vi "WHD_VEten_0.1.1_WS_BIDIR.vi"() -> ()   [LabVIEW 2015]
uses:
  <vilib>/LabVIEW Targets/FPGA/cRIO/shared/nicrio_ModuleControls/nicrio_cRIO-9234_DataRatesRing2.ctl
  <vilib>/RTwatchdog.llb/Watchdog expiration actions.ctl
  <vilib>/userDefined/High Color/nirio_resource_hc.ctl
  <vilib>/FPGAPlugInAG/cRIO-9031/niLvFpga_Open_cRIO-9031.vi
  <vilib>/Utility/error.llb/Error Cluster From Error Code.vi
  <vilib>/rvi/errors/niLvFpgaAdjustHostInterfaceError.vi
  <vilib>/Utility/file.llb/Write Delimited Spreadsheet (string).vi
  <vilib>/FPGAPlugInAG/cRIO-9031/niLvFpga_Run_cRIO-9031.vi
  <vilib>/rvi/interface/common/niFpgaWaitOnOcc.vi
  <vilib>/FPGAPlugInAG/cRIO-9031/niLvFpga_Reset_cRIO-9031.vi
  <vilib>/FPGAPlugInAG/cRIO-9031/niLvFpga_Close_cRIO-9031.vi
  <vilib>/rvi/interface/nirviOpenFPGA/nirviOpenFPGA.xnode
  FPGA Bitfiles/W&RDEuskotrenViz_FPGATarget2_FPGA8a2wsBIdirec_eiRvK+Hs3vw.lvbitx
  <vilib>/rvi/interface/nirviReadWriteControl/nirviReadWriteControl.xnode
  <vilib>/rvi/interface/nirviMethod/nirviMethod.xnode
  <vilib>/rvi/interface/nirviCloseFPGA/nirviCloseFPGA.xnode
  <vilib>/NI_Real-Time Target Support.lvlib
  <vilib>/rvi/errors/niLvFpgaMergeErrorWithErrorCode.vi
  <vilib>/nisyscfg/nisyscfg.lvlib
  AURA_Wheel/Json2Labv.lvlib
  AURA_Wheel/AuraWheelAPI/AuraWheel.lvlib
  NiFpgaLv.dll
  <vilib>/FPGAPlugInAG/cRIO-9031/niLvFpga_ConfigureFifo_cRIO-9031.vi
  <vilib>/FPGAPlugInAG/cRIO-9031/niLvFpga_StartFifo_cRIO-9031.vi
  <vilib>/FPGAPlugInAG/cRIO-9031/niLvFpga_ReadFifo_cRIO-9031.vi
  <vilib>/FPGAPlugInAG/cRIO-9031/niLvFpga_StopFifo_cRIO-9031.vi
panel:
  out "Direccion 0?":bool
  out "Boton Adquirir?":bool
  out "RuedaDetectada2?":bool=TRUE
  out "RuedaDetectada1?":bool=TRUE
  in  "Timeout ruedas":dbl
  in  "Borrar archivos\nadquisicion con error":bool
  in  "Able watchdog?":bool
  in  "Reset watchdog?":bool
  in  "Leer config RFID NEM":bool
  in  "bytes to read":i32
  in  "DeviceAddress":u8
  in  "timeout ms (60000)":i32
  in  "Max archivos":u32=2
  in  "Bytes libre despues de borrar":u32=2
  in  "Bytes min libre":u32=2
  in  "Nº de acelerómetros":i32
  in  "Nº inductivos":i32
  in  "Offset_rueda WS 1":fxp<+/-,24,-4>=0.004999998956918716 format="%.27g"
  out "TAGs_AURAwheel":string[][](array[string])
  out "Plataformas?":bool
  out "Nº Ejes":i32[](array[numeric])
  out "Nº UTs":i32
  out "it-read-LR6":i32[](array[numeric])
  out "it-LR6":i32
  out "RFID_LR6_Error":errorcluster
  out "Series_flota":string[](array[string])
  out "Tabla_flota":string[][](array[string])
  out "Puntos medios de las ventanas":dbl[][](array[numeric])
  out "configuration file path":path=path "c:/Parametros.cfg"
  in  "IP synchr":string
  out "data":cluster{"status":string}
  out "confRFID":path=path "c:/RFID/TAGS.csv"
  out "TAGS leidos":path=path "c:/RFID/TAGS.csv"
  in  "Use Aura?":bool
  in  "Parametros AuraWheel":string[](array[string])
  in  "Parámetros acelerómetros":dbl[](array[numeric])
  in  "Tiempo de adquisicion":dbl=10.0
  in  "Adquirir":bool
  out "Fin":bool
  out "Contador":i32=1
  out "Path TEST":path=path "c:/TEST"
  out "Fallo fotocelula":bool
  out "Path_Borrar":path=path "c:/Trenes"
  out "Longitud de la unidad":dbl
  out "Aviso no detección":string
  out "Time to Acquire Block (ms)":i32
  out "Distancia de acelerómetros":dbl[](array[numeric])
  out "Block Size":u32
  out "Distancias generales":dbl[](array[numeric])
  in  "Reset del controlador":bool
  in  "Configuración":bool
  in  "Parar la aplicación":bool
  out "RFID":bool=TRUE
  out "date/time string":string
  out "Timeout ruedas":bool
  out "Tiempo":dbl
  out "Inicio pasada":timestamp
  out "Ultimo TEST":timestamp
  out "Fuente":bool=TRUE
  out "Estado":string
  out "RFID_ID":refnum<k5>
  out "DC OK":string
  out "Aviso temperatura":string
  in  "Tab Control":T1(tab)=enum."Parámetros"
  out "V (m/s)":dbl
  out "Temperatura (ºC)":dbl
  out "Max RMS Ruedas":dbl[][](array[numeric])
  out "result":bool
  out "TAGs":string[](array[string])
  out "Parar":bool
  out "TAGs LR6":string[](array[string])
  out "TAGs HEX":string[](array[string])
  out "Waveform Graph 2":sgl[](graph)
  out "Waveform Graph":sgl[][](graph)
  out "Nombre de archivo":path[](array[path])
  out "Tiempo de paso (s)":dbl
  out "Tiempo extra de adquisición (s)":dbl
  out "Número de ejes detectados":i32
  out "Buffer Underflow":bool
  out "Buffer Overflow":bool
  out "Disco Duro Disponible (bytes)":i64
  out "created path":path
  out "Nº Ruedas 1":i32
  out "NºRuedas 2":i32
  out "deleted portion":sgl[](array[numeric])
  out "deleted portion 2":sgl[](array[numeric])
  out "Ejes_convoy":i32
  out "Archivo\nvalido?":bool
  out "T fuera rango":bool
  in  "Frecuencia de muestreo (Hz)":dbl=25600.0
  in  "Escaneos de la FIFO por canal":u32=5000
  in  "Tiempo extra al detector de paso (s)":dbl=1.0
  in  "dt RMS":dbl=256.0
  in  "Frecuencia de muestreo y módulo CRIO":T2=2 items=["51.200 kS/s (NI 9234)"=1, "25.600 kS/s (NI 9234)"=2, "17.067 kS/s (NI 9234)"=3, "12.800 kS/s (NI 9234)"=4, "10.240 kS/s (NI 9234)"=5, "8.533 kS/s (NI 9234)"=6, "7.314 kS/s (NI 9234)"=7, "6.400 kS/s (NI 9234)"=8, "5.689 kS/s (NI 9234)"=9, "5.120 kS/s (NI 9234)"=10, "4.654 kS/s (NI 9234)"=11, "4.267 kS/s (NI 9234)"=12, "3.938 kS/s (NI 9234)"=13, "3.657 kS/s (NI 9234)"=14, "3.413 kS/s (NI 9234)"=15, "3.200 kS/s (NI 9234)"=16, "3.012 kS/s (NI 9234)"=17, "2.845 kS/s (NI 9234)"=18, "2.695 kS/s (NI 9234)"=19, "2.560 kS/s (NI 9234)"=20, "2.438 kS/s (NI 9234)"=21, "2.328 kS/s (NI 9234)"=22, "2.226 kS/s (NI 9234)"=23, "2.133 kS/s (NI 9234)"=24, "2.048 kS/s (NI 9234)"=25, "1.969 kS/s (NI 9234)"=26, "1.896 kS/s (NI 9234)"=27, "1.829 kS/s (NI 9234)"=28, "1.765 kS/s (NI 9234)"=29, "1.707 kS/s (NI 9234)"=30, "1.652 kS/s (NI 9234)"=31]
  in  "Puerto RFID":u16=2189
  in  "IP RFID":string="192.168.106.99"
  in  "Offset_rueda WS 2":fxp<+/-,24,-4>=0.004999998956918716 format="%.27g"
  in  "Count(mSec)":u32=2
  in  "LR6 IP address":string="192.168.106.94"
  in  "Port LR6":u16=2001
  in  "RFID NEM on?":bool
  in  "RFID LR6 on?":bool
  in  "Canal cero WS1?":bool
  in  "Canal cero WS2":bool
  out "Parámetros":bool=TRUE
  out "Distacias y medidas de dispositivos":bool=TRUE
  out "RFID_Error":errorcluster
  out "error FPGA":errorcluster
  out "error manipulacion archivos":errorcluster
  out "Unidades y ejes":bool=TRUE
  out "RFID":bool=TRUE
  out "error AURA":errorcluster
  out "Response headers":string
  out "Numeric 3":i32
  in  "Digital?":bool=TRUE
  out "Bucle Espera":i32
  out "Watchdog config":T3={"reset"=FALSE, "occurrence"=FALSE, "trigger protocol"=enum."active high", "trigger line"=enum."none", "disable watchdog on VI exit"=TRUE}
  # "Funciona?"
  # "Última detección de unidad"
  # "Error!!"
  # "Estado de la memoria"
  # "Parámetros de muestreo"
  # "Parámetros de adquisición"
  # "Parámetros de procesado"
  # "Cambio Fecha y Hora"
  # "Cargar datos de configuración"
  # "Errores!!"
  # "WRD_MEX\nWRD_ZAR"
  # "0 tagMexInit\n1 tagMexFin\n\n0 tag1\n1 tag2"
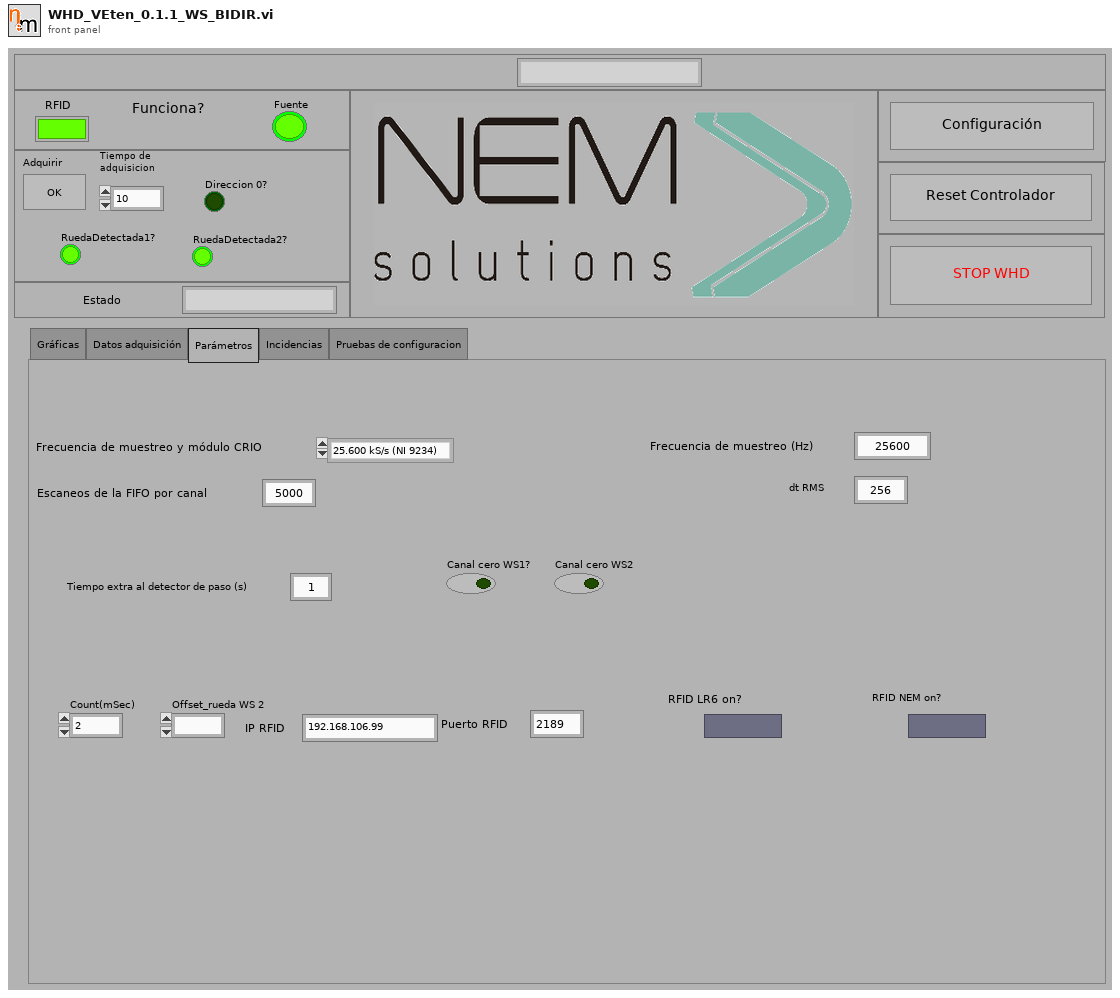
[diagram p1: front panel]
types:
  T1 = enum32{"Gráficas", "Datos adquisición", "Parámetros", "Incidencias", "Pruebas de configuracion"}
  T2 = typedef "nicrio_cRIO-9234_DataRatesRing2.ctl" = u8
  T3 = typedef "Watchdog expiration actions.ctl" = cluster{"reset":bool, "occurrence":bool, "trigger protocol":enum16{"active high", "active low", "open collector"}, "trigger line":enum16{"none", "line 0", "line 1", "line 2", "line 3", "line 4", "line 5", "line 6", "line 7", "SMB line 0"}, "disable watchdog on VI exit":bool}
  T4 = typedef "nirio_resource_hc.ctl" = tag
  T5 = enum16{"Standard", "Buffered", "CRLF", "Immediate"}
  T6 = enum16{"open", "replace", "create", "open or create", "replace or create", "replace or create with confirmation"}
  T7 = enum16{"big-endian, network order", "native, host order", "little-endian"}
  T8 = cluster{"error IO":errorcluster, bool[], u32[], string[], dbl[]}
  T9 = cluster{"g_ts":dbl, "p_sp":dbl, "p_tp":dbl, "p_tg":cluster{"tg_n":dbl, "tg_t":string}[], "p_ax":cluster{"ax_n":dbl, "ax_sp":dbl, "ax_wh":cluster{"wh_p":dbl, "wh_a1":dbl, "wh_a2":dbl, "wh_a3":dbl, "wh_a4":dbl}[]}[]}
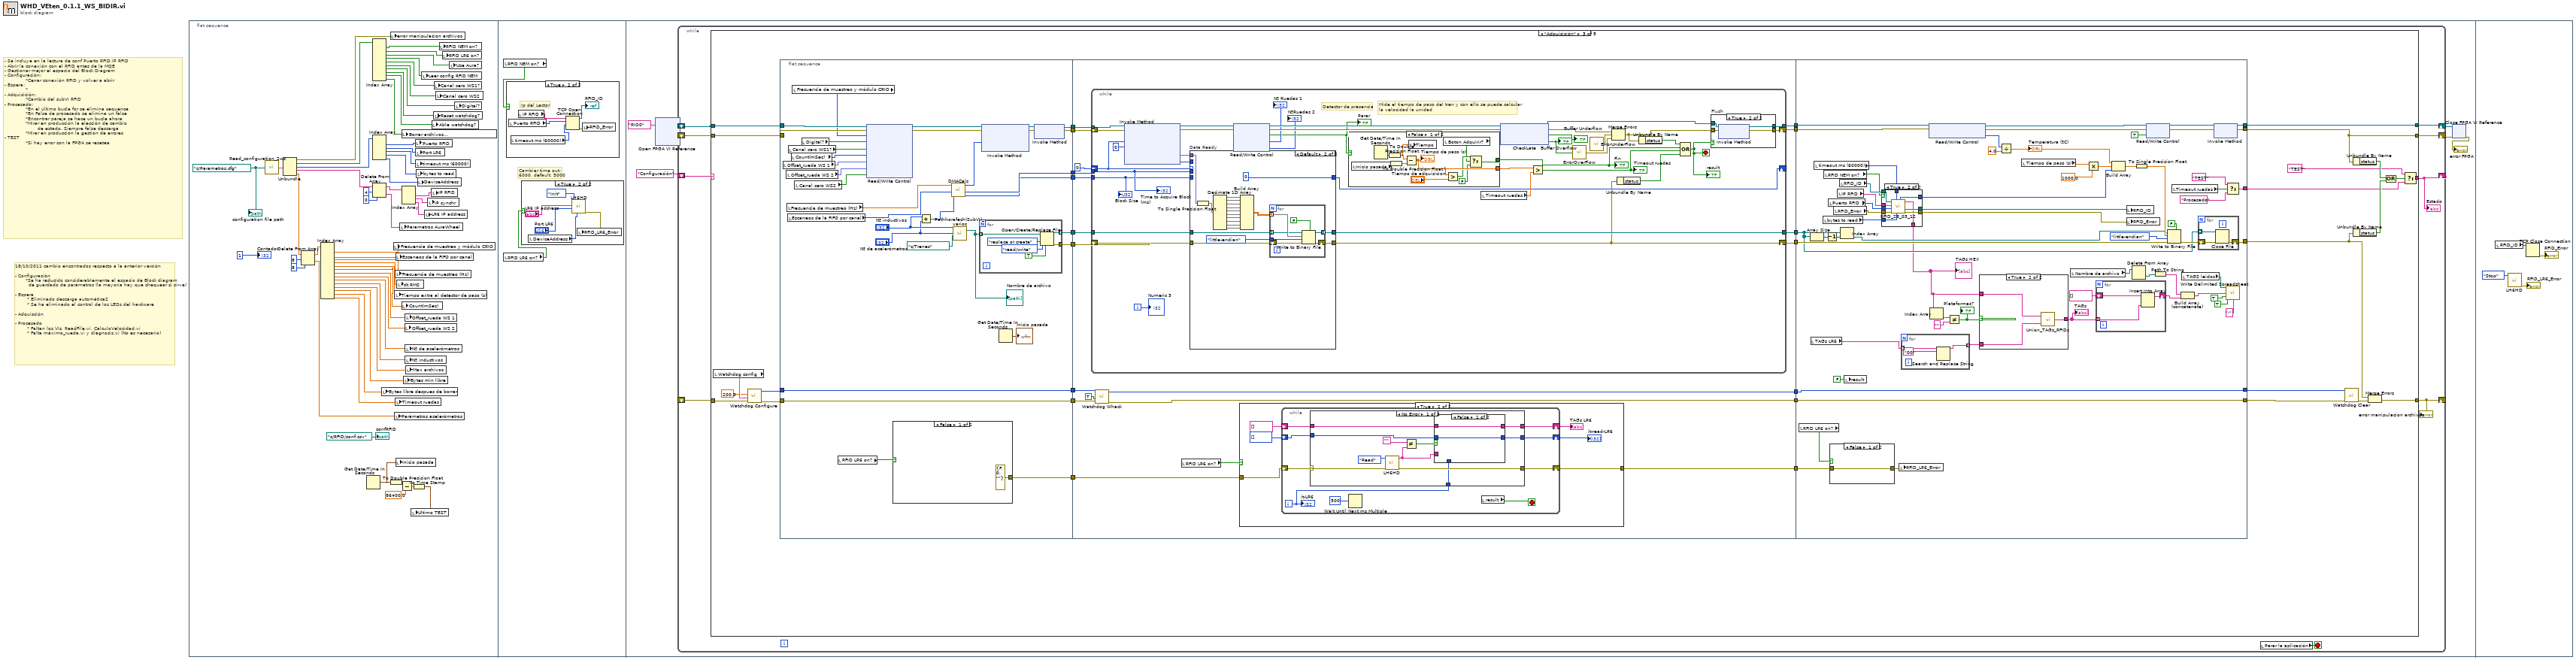
[diagram p0: block diagram]
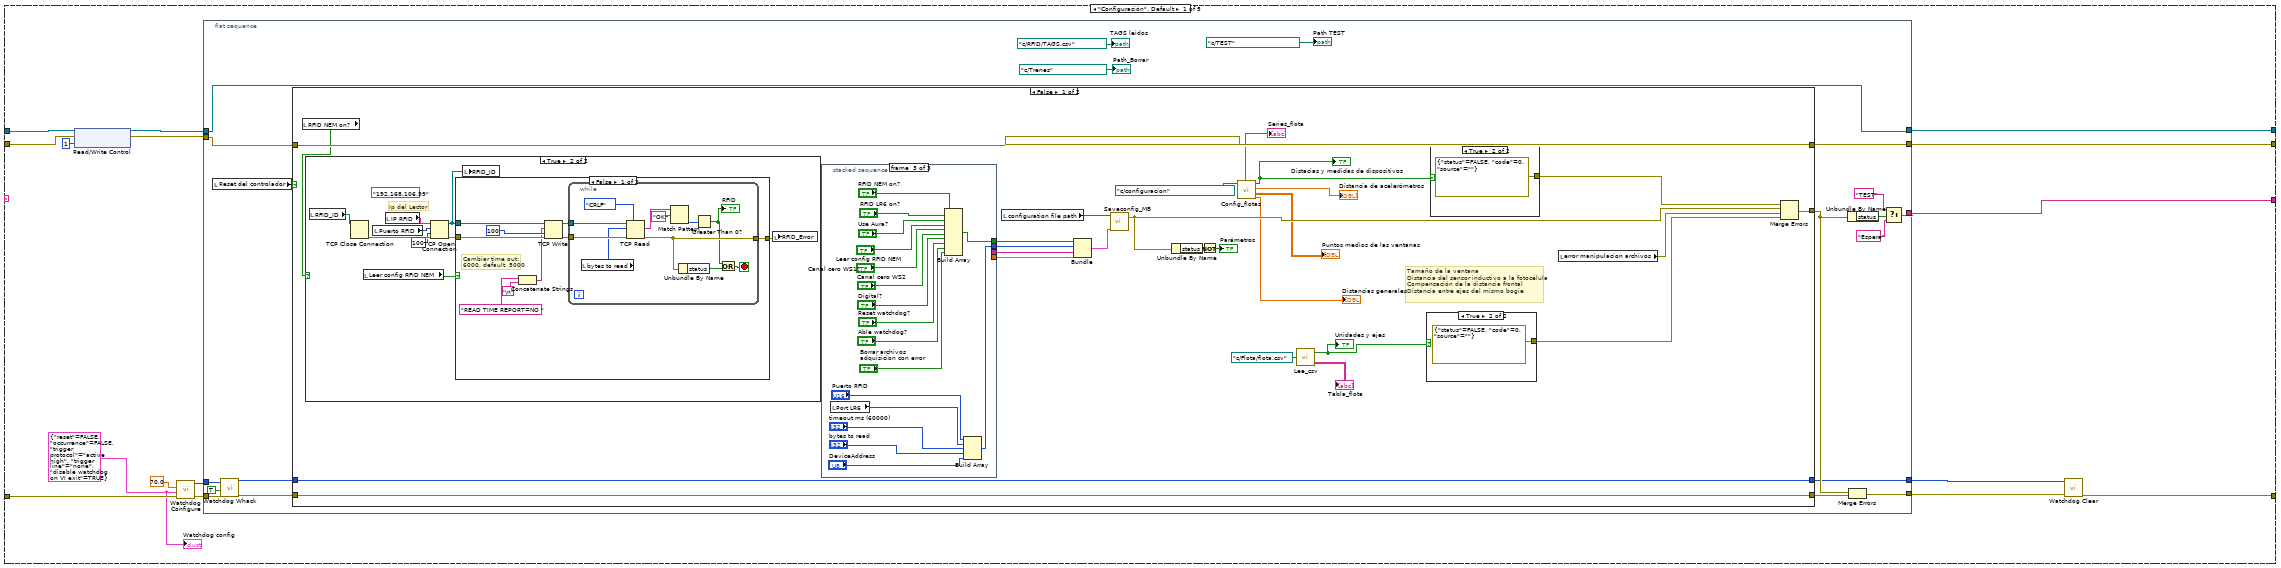
[diagram p4: hidden frame]
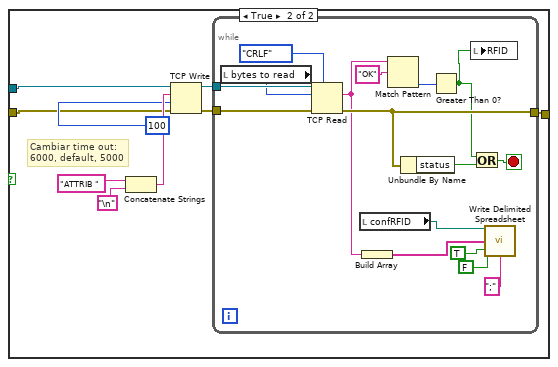
[diagram p6: hidden frame]
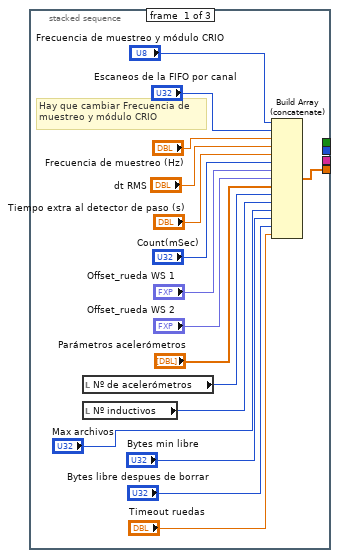
[diagram p7: hidden frame]
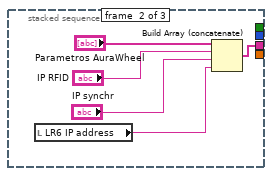
[diagram p8: hidden frame]
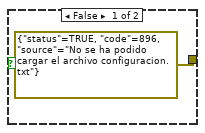
[diagram p9: hidden frame]
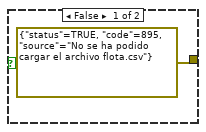
[diagram p10: hidden frame]
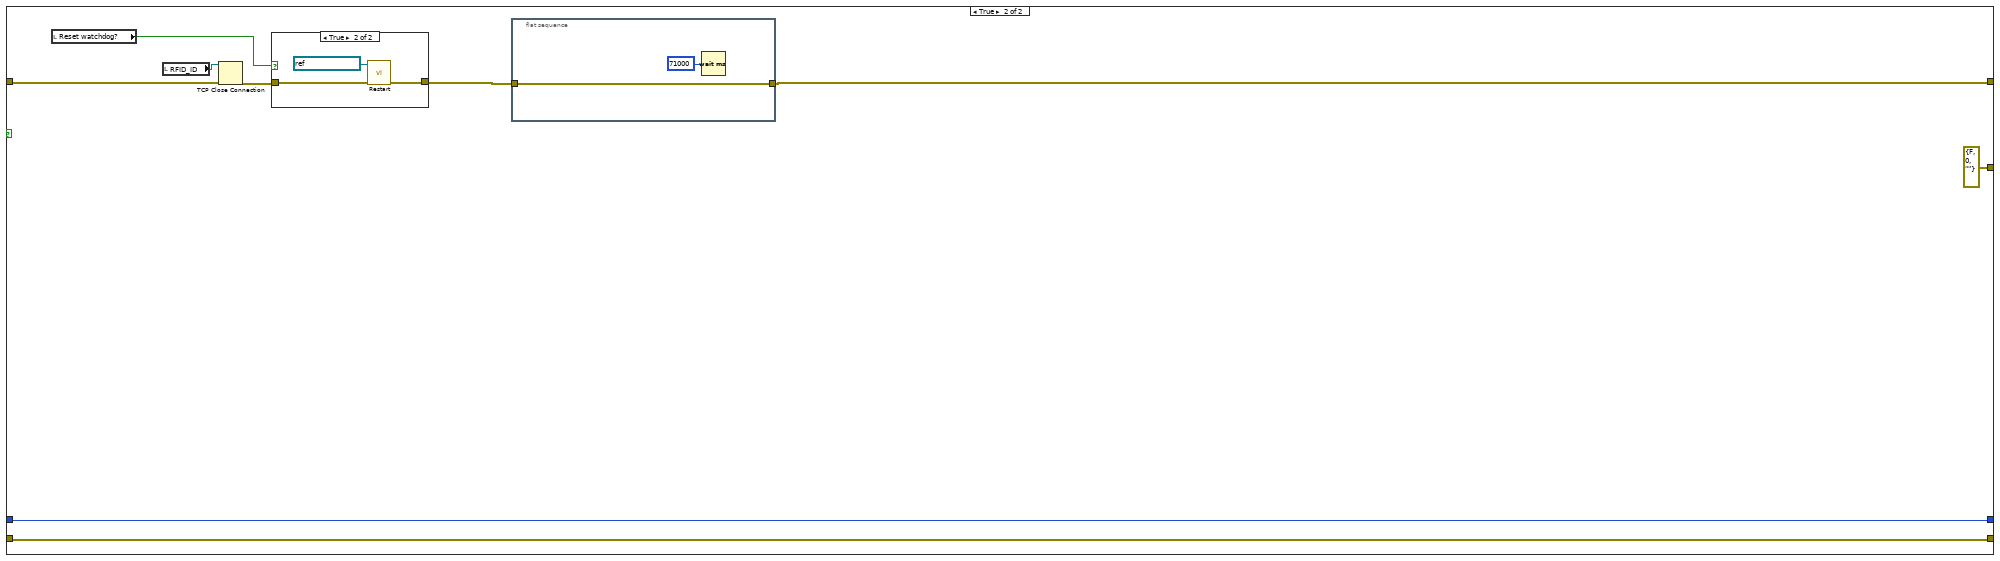
[diagram p11: hidden frame]
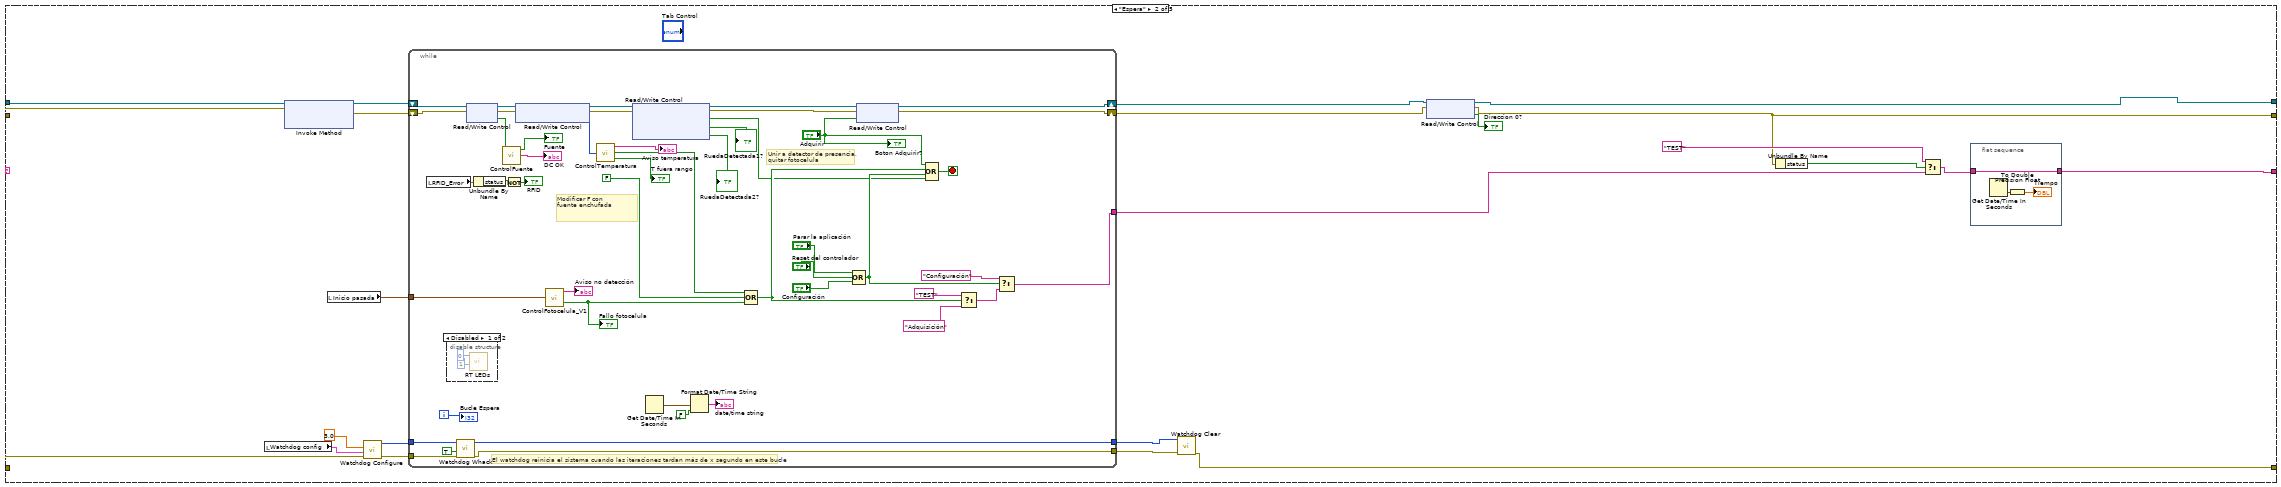
[diagram p13: hidden frame]
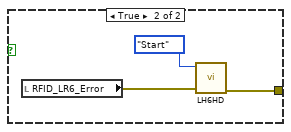
[diagram p15: hidden frame]
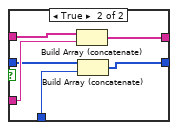
[diagram p17: hidden frame]
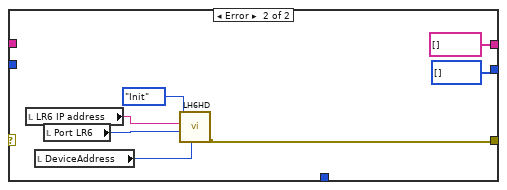
[diagram p18: hidden frame]
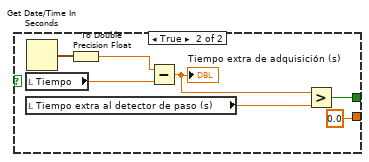
[diagram p19: hidden frame]
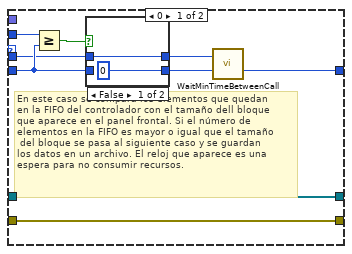
[diagram p20: hidden frame]
diagram:
  # "18/10/2011 cambio encontrados respecto a la anterior versión\n\n- Configuración\n       *Se ha reducido considerablemente el espacio de Block diagram\n         de guardado de parámetros (la mayoría hay que chequear si sirve)\n\n- Espera\n        * Eliminado descarga automática2\n        * Se ha eliminado el control de los LEDs del hardware\n       \n- Adquisción\n\n- Procesado\n        * Faltan los VIs, ReadFile.vi, CalculoVelocidad.vi\n        * Falta máximo_rueda.vi y diagnosis.vi (No es necesario)"
  # "- Se incluye en la lectura de conf Puerto RFID,IP RFID\n- Abrir la conexión con el RFID antes de la MQE\n- Gestionar mejor el espacio del Block Diagram\n- Configuración:\n              *Cerrar conexión RFID y volver a abrir\n- Espera:\n              *\n- Adquisición:\n              *Cambio del subVI RFID\n- Procesado:\n              *En el último bucle for se elimina sequence\n              *En False de procesado se elimina un false\n              *Encontrar pareja se hace un bucle ahora\n              *Mirar en producción la elección de cambio\n                      de estado. Siempre false descarga \n              *Mirar en produccion la gestion de errores\n- TEST\n              *Si hay error con la FPGA se resetea"
  n1 = flat-sequence {
    frame #0 {
      w38 = path "c:/Parametros.cfg" ("configuration file path")
      n2 = call "Read_configuration_2ws.vi"("configuration file path"=w38) -> ("output cluster"=w37:T8)
      n3 = Unbundle(w37) -> ("error IO"=w42:errorcluster, w41:bool[], w40:u32[], w29:string[], w35:dbl[])
      n4 = Delete From Array(array=w35, length=8, index=8) -> (deleted portion=w31:dbl[], array with subset deleted=w34:dbl[])
      n5 = Index Array(array=w34) -> (element #1=w49:dbl, element #2=w48:dbl, element #3=w47:dbl, element #4=w46:dbl, element #5=w45:dbl, element #6=w19:dbl, element #7=w18:dbl, element #8=w1:dbl, element #9=w17:dbl, element #10=w16:dbl, element #11=w15:dbl, element #12=w14:dbl, element #13=w13:dbl, element #14=w2:dbl)  [unwired: 14 in]
      n6 = Get Date/Time In Seconds() -> (seconds since 1Jan1904=w51:timestamp)
      n7 = Index Array(array=w41) -> (element #1=w44:bool, element #2=w43:bool, element #3=w30:bool, element #4=w9:bool, element #5=w8:bool, element #6=w7:bool, element #7=w6:bool, element #8=w5:bool, element #9=w4:bool, element #10=w3:bool)  [unwired: 10 in]
      n8 = Index Array(array=w40) -> (element #1=w36:u32, element #2=w20:u32, element #3=w12:u32, element #4=w11:u32, element #5=w10:u32)  [unwired: 5 in]
      n9 = Delete From Array(array=w29, length=4, index=0) -> (deleted portion=w23:string[], array with subset deleted=w28:string[])
      n10 = local write "Bytes libre despues de borrar"(w13) -> ()
      n11 = To Double Precision Float(number=w51) -> (double precision float=w53:dbl)
      n12 = local write "error manipulacion archivos"(w42) -> ()
      n13 = local write "Frecuencia de muestreo y módulo CRIO"(w49) -> ()
      n14 = local write "Parámetros acelerómetros"(w31) -> ()
      n15 = local write "Tiempo extra al detector de paso (s)"(w45) -> ()
      n16 = local write "Frecuencia de muestreo (Hz)"(w47) -> ()
      n17 = local write "Timeout ruedas"(w2) -> ()
      n18 = local write "Escaneos de la FIFO por canal"(w48) -> ()
      n19 = local write "Inicio pasada"(w51) -> ()
      n20 = local write "dt RMS"(w46) -> ()
      n21 = local write "Parametros AuraWheel"(w23) -> ()
      n22 = Subtract(x=w53, y=86400.0) -> (x-y=w52:dbl)
      n23 = local write "Borrar archivos\nadquisicion con error"(w3) -> ()
      n24 = Index Array(array=w28) -> (element #1=w22:string, element #2=w24:string, element #3=w21:string)  [unwired: 3 in]
      n25 = local write "Count(mSec)"(w19) -> ()
      n26 = local write "Bytes min libre"(w14) -> ()
      n27 = local write "Offset_rueda WS 2"(w1) -> ()
      n28 = local write "Offset_rueda WS 1"(w18) -> ()
      n29 = local write "Nº de acelerómetros"(w17) -> ()
      n30 = local write "Nº inductivos"(w16) -> ()
      n31 = local write "Max archivos"(w15) -> ()
      n32 = To Time Stamp(1:w52) -> (0:w50:timestamp)
      n33 = local write "Ultimo TEST"(w50) -> ()
      n34 = local write "Puerto RFID"(w36) -> ()
      n35 = local write "Port LR6"(w20) -> ()
      n36 = local write "timeout ms (60000)"(w12) -> ()
      n37 = local write "bytes to read"(w11) -> ()
      n38 = local write "DeviceAddress"(w10) -> ()
      n39 = local write "Leer config RFID NEM"(w9) -> ()
      n40 = local write "LR6 IP address"(w21) -> ()
      n41 = local write "IP synchr"(w24) -> ()
      n42 = local write "IP RFID"(w22) -> ()
      n43 = local write "Able watchdog?"(w4) -> ()
      n44 = local write "Reset watchdog?"(w5) -> ()
      n45 = local write "Canal cero WS1?"(w8) -> ()
      n46 = local write "Canal cero WS2"(w7) -> ()
      n47 = local write "RFID NEM on?"(w44) -> ()
      n48 = local write "RFID LR6 on?"(w43) -> ()
      n49 = local write "Use Aura?"(w30) -> ()
      n50 = local write "Digital?"(w6) -> ()
      "Contador" <- 1
      "confRFID" <- path "c:/RFID/conf.csv" ("file path (use dialog)")
      "configuration file path" <- w38
    }
    frame #1 {
      # "Cambiar time out:\n6000, default, 5000"
      n51 = local read "RFID NEM on?"() -> (w56:bool)
      n52 = local read "RFID LR6 on?"() -> (w55:bool)
      n53 = case shown="True" w56 {
        frame False {
        }
        frame True {
          # "Ip del Lector"
          n54 = local read "Puerto RFID"() -> (w64:u16)
          n55 = local read "timeout ms (60000)"() -> (w62:i32)
          n56 = local read "IP RFID"() -> (w65:string)
          n57 = TCP Open Connection(address=w65, remote port or service name=w64, timeout ms (60000)=w62) -> (connection ID=→"RFID_ID":refnum<k5>, error out=w63:errorcluster)  [unwired: 1 in, 1 out]
          n58 = local write "RFID_Error"(w63) -> ()
        }
      }
      n59 = case shown="True" w55 {
        frame False {
        }
        frame True {
          n60 = local read "DeviceAddress"() -> (w57:u8)
          n61 = call "LH6HD.vi"("DeviceAddress"=w57, "Reader Port"="Port LR6", "IP Address"="LR6 IP address", "Action"=enum16{"Init", "Start", "Read", "Stop", "Exit"}."Init") -> ("error out"=w61:errorcluster)  [unwired: 6 in, 1 out]
          n62 = local write "RFID_LR6_Error"(w61) -> ()
        }
      }
    }
    frame #2 {
      n63 = xnode "Open FPGA VI Reference"("resource name"=T4 "RIO0") -> ("FPGA VI Reference Out"=w73:refnum<k20>, "error out"=w72:errorcluster)  [unwired: 1 in]
      n64 = while {
        shift-right: [w77] -> _
        shift-left: "Configuración" -> [w82]
        shift-right: [w75] -> w69
        shift-left: w73 -> [w81]
        shift-right: [w74] -> w68
        shift-left: w72 -> [w80]
        shift-right: [w79] -> _
        shift-left: _ -> [w78]
        stop <- w76 stop-if-true
        n65 = case shown="\"Adquisición\"" w82 {
          tunnel: [w97 w269 w345 w676 w917] -> w77
          tunnel: [w96 w257 w359 w684 w916] -> w75
          tunnel: [w98 w256 w360 w671 w914] -> w74
          tunnel: w81 -> [w88 w274 w367 w684 w916]
          tunnel: w80 -> [w86 w272 w366 w671 w915]
          tunnel: [w89 w263 w357 w674 w904] -> w79
          tunnel: w78 -> [w95 w268 w341 w670 w909]
          frame "Configuración", Default {
            w83 = T3 {"reset"=FALSE, "occurrence"=FALSE, "trigger protocol"=enum."active high", "trigger line"=enum."none", "disable watchdog on VI exit"=TRUE} ("expiration actions")
            n66 = xnode "Read/Write Control"("FPGA VI Reference In"=w88, "error in"=w86, "Cycles to Filter"=u16 1) -> ("FPGA VI Reference Out"=w87:refnum<k20>, "error out"=w85:errorcluster)
            n67 = call <vilib>:"Watchdog Configure.vi"("error in (no error)"=w95, "expiration actions"=w83, "timeout (1 sec)"=70.0) -> ("error out"=w92:errorcluster, "watchdogID"=w93:u64)  [unwired: 1 in, 2 out]
            n68 = flat-sequence {
              tunnel: [w109] -> w98
              tunnel: [w117] -> w97
              tunnel: w87 -> [w110]
              tunnel: [w110] -> w96
              tunnel: [w112] -> w90
              tunnel: w85 -> [w107]
              tunnel: w93 -> [w105]
              tunnel: w92 -> [w104]
              tunnel: [w102] -> w91
              frame #0 {
                n69 = local read "Reset del controlador"() -> (w106:bool)
                n70 = call <vilib>:"Watchdog Whack.vi"("error in (no error)"=w104, "reset watchdog after expire? (F)"=TRUE, "watchdogID in"=w105) -> ("error out"=w100:errorcluster, "watchdogID out"=w101:u64)  [unwired: 2 in, 1 out]
                n71 = case shown="False" w106 {
                  tunnel: w107 -> [w144 w247]
                  tunnel: [w144 w246] -> w109
                  tunnel: [w130 errorcluster {"status"=FALSE, "code"=0, "source"=""} ("error IO")] -> w108
                  tunnel: [w122 w245] -> w102
                  tunnel: w101 -> [w122 w245]
                  tunnel: w100 -> [w121 w244]
                  tunnel: [w121 w244] -> w99
                  frame False {
                    # "Tamaño de la ventana\nDistancia del sensor inductivo a la fotocélula\nCompensación de la distancia frontal\nDistancia entre ejes del mismo bogie"
                    n72 = local read "RFID NEM on?"() -> (w120:bool)
                    n73 = case shown="True" w120 {
                      frame False {
                      }
                      frame True {
                        (unwired) "192.168.106.99" ("address")
                        # "Ip del Lector"
                        n74 = local read "RFID_ID"() -> (w152:refnum<k5>)
                        n75 = TCP Close Connection(connection ID=w152) -> (error out=w153:errorcluster)  [unwired: 2 in, 1 out]
                        n76 = local read "Leer config RFID NEM"() -> (w145:bool)
                        n77 = local read "Puerto RFID"() -> (w150:u16)
                        n78 = local read "IP RFID"() -> (w149:string)
                        n79 = TCP Open Connection(address=w149, remote port or service name=w150, timeout ms (60000)=100, error in (no error)=w153) -> (connection ID=w151:refnum<k5>, error out=w146:errorcluster)  [unwired: 1 out]
                        n80 = case shown="False" w145 {
                          tunnel: w151 -> [w162 w176]
                          tunnel: [w160 w174] -> w147
                          tunnel: w146 -> [w157 w175]
                          frame False {
                            # "Cambiar time out:\n6000, default, 5000"
                            n81 = Concatenate Strings("READ TIME REPORT=NO " ("data in"), "\n") -> (w154:string)
                            n82 = TCP Write(connection ID=w162, data in=w154, error in (no error)=w157, 9:100 ("timeout ms (25000)")) -> (connection ID out=w158:refnum<k5>, error out=w159:errorcluster)  [unwired: 1 out]
                            n83 = while {
                              tunnel: w159 -> [w172]
                              tunnel: w158 -> [w171]
                              tunnel: [w170] -> w160
                              stop <- w167 stop-if-true
                              n84 = local read "bytes to read"() -> (w163:i32)
                              n85 = TCP Read(connection ID=w171, bytes to read=w163, error in (no error)=w172, 7:T5."CRLF" ("mode (standard)")) -> (data out=w165:string, error out=w170:errorcluster)  [unwired: 1 in, 1 out]
                              n86 = Match Pattern(string=w165, regular expression="OK") -> (offset past match=w168:i32)  [unwired: 4 out]
                              n87 = Unbundle By Name(w170) -> ("status"=w166:bool)
                              n88 = Greater Than 0?(x=w168) -> (x > 0?=w164:bool)
                              "RFID" <- w164
                              n89 = Or(x=w164, y=w166) -> (x .or. y?=w167:bool)
                            }
                          }
                          frame True {
                            # "Cambiar time out:\n6000, default, 5000"
                            n90 = Concatenate Strings("ATTRIB " ("data in"), "\n") -> (w182:string)
                            n91 = TCP Write(connection ID=w176, data in=w182, error in (no error)=w175, 9:100 ("timeout ms (25000)")) -> (connection ID out=w179:refnum<k5>, error out=w178:errorcluster)  [unwired: 1 out]
                            n92 = while {
                              tunnel: w178 -> [w197]
                              tunnel: w179 -> [w196]
                              tunnel: [w195] -> w174
                              stop <- w192 stop-if-true
                              n93 = local read "bytes to read"() -> (w183:i32)
                              n94 = TCP Read(connection ID=w196, bytes to read=w183, error in (no error)=w197, 7:T5."CRLF" ("mode (standard)")) -> (data out=w186:string, error out=w195:errorcluster)  [unwired: 1 in, 1 out]
                              n95 = local read "confRFID"() -> (w185:path)
                              n96 = Build Array(w186) -> (w184:string[])
                              n97 = Match Pattern(string=w186, regular expression="OK") -> (offset past match=w193:i32)  [unwired: 4 out]
                              n98 = Unbundle By Name(w195) -> ("status"=w191:bool)
                              n99 = Greater Than 0?(x=w193) -> (x > 0?=w190:bool)
                              n100 = local write "RFID"(w190) -> ()
                              n101 = Or(x=w190, y=w191) -> (x .or. y?=w192:bool)
                              n102 = call-poly <vilib>:"Write Delimited Spreadsheet.vi"("file path (dialog if empty)"=w185, "1D data"=w184, "append to file? (F)"=FALSE ("transpose? (no:F)"), "transpose? (F)"=TRUE ("append to file? (new file:F)"), "delimiter (\\t)"=";" ("delimiter (\\t)")) -> ()  [unwired: 9 in, 2 out]
                            }
                          }
                        }
                        n103 = local write "RFID_ID"(w151) -> ()
                        n104 = local write "RFID_Error"(w147) -> ()
                      }
                    }
                    n105 = stacked-sequence {
                      tunnel: [w210 _ _] -> w134
                      tunnel: [_ w219 _] -> w133
                      tunnel: [_ _ w233] -> w135
                      tunnel: [_ _ w232] -> w136
                      frame #0 {
                        # "Hay que cambiar Frecuencia de\nmuestreo y módulo CRIO"
                        n106 = local read "Nº de acelerómetros"() -> (w204:i32)
                        n107 = local read "Nº inductivos"() -> (w203:i32)
                        n108 = Build Array (concatenate)("Frecuencia de muestreo y módulo CRIO", "Escaneos de la FIFO por canal", "Frecuencia de muestreo (Hz)", "dt RMS", "Tiempo extra al detector de paso (s)", "Count(mSec)", "Offset_rueda WS 1", "Offset_rueda WS 2", "Parámetros acelerómetros", w204, w203, "Max archivos", "Bytes min libre", "Bytes libre despues de borrar", "Timeout ruedas") -> (w210:dbl[])
                      }
                      frame #1 {
                        n109 = local read "LR6 IP address"() -> (w215:string)
                        n110 = Build Array (concatenate)("Parametros AuraWheel", "IP RFID", "IP synchr", w215) -> (w219:string[])
                      }
                      frame #2 {
                        n111 = local read "Port LR6"() -> (w229:u16)
                        n112 = Build Array("RFID NEM on?", "RFID LR6 on?", "Use Aura?", "Leer config RFID NEM", "Canal cero WS1?", "Canal cero WS2", "Digital?", "Reset watchdog?", "Able watchdog?", "Borrar archivos\nadquisicion con error") -> (w232:bool[])
                        n113 = Build Array("Puerto RFID", w229, "timeout ms (60000)", "bytes to read", "DeviceAddress") -> (w233:i32[])
                      }
                    }
                    n114 = local read "configuration file path"() -> (w131:path)
                    n115 = Bundle(w136, w135, w133, w134) -> (w132:cluster{bool[], i32[], string[], dbl[]})  [unwired: 1 in]
                    n116 = call "Saveconfig_MB.vi"("configuration file path"=w131, "Configuracion"=w132) -> ("error out"=w139:errorcluster)  [unwired: 4 in]
                    n117 = Unbundle By Name(w139) -> ("status"=w140:bool)
                    n118 = Not(x=w140) -> (.not. x?=→"Parámetros":bool)
                    n119 = call "Config_flotas.vi"("file path (dialog if empty)"=path "c:/configuracion") -> ("Distancias generales"=→"Distancias generales":dbl[], "Puntos medios de las ventanas"=→"Puntos medios de las ventanas":dbl[][], "Distancia de acelerómetros"=→"Distancia de acelerómetros":dbl[], "Distacias y medidas de dispositivos"=w129:bool, "Series_flota"=→"Series_flota":string[])  [unwired: 3 in]
                    "Distacias y medidas de dispositivos" <- w129
                    n120 = call "Lee_csv.vi"("Path"=path "c:/Flota/flota.csv") -> ("Tabla_flota"=→"Tabla_flota":string[][], "Lectura_OK?"=w126:bool)
                    "Unidades y ejes" <- w126
                    n121 = case shown="True" w126 {
                      tunnel: [errorcluster {"status"=TRUE, "code"=895, "source"="No se ha podido cargar el archivo flota.csv"} ("error out") errorcluster {"status"=FALSE, "code"=0, "source"=""} ("error out")] -> w137
                      frame False {
                      }
                      frame True {
                      }
                    }
                    n122 = case shown="True" w129 {
                      tunnel: [errorcluster {"status"=TRUE, "code"=896, "source"="No se ha podido cargar el archivo configuracion.txt"} ("error out") errorcluster {"status"=FALSE, "code"=0, "source"=""} ("error out")] -> w142
                      frame False {
                      }
                      frame True {
                      }
                    }
                    n123 = local read "error manipulacion archivos"() -> (w138:errorcluster)
                    n124 = Merge Errors(w142, w139, w138, w137) -> (w130:errorcluster)
                  }
                  frame True {
                    n125 = local read "Reset watchdog?"() -> (w241:bool)
                    n126 = local read "RFID_ID"() -> (w249:refnum<k5>)
                    n127 = TCP Close Connection(connection ID=w249, error in (no error)=w247) -> (error out=w243:errorcluster)  [unwired: 2 out]
                    n128 = case shown="True" w241 {
                      tunnel: w243 -> [w250 w253]
                      tunnel: [w250 w252] -> w242
                      frame False {
                      }
                      frame True {
                        n129 = call <vilib>:"Restart.vi"("error in (no error)"=w253, "Session in"=refnum<k21> "localhost") -> ("error out"=w252:errorcluster)  [unwired: 7 in, 2 out]
                      }
                    }
                    n130 = flat-sequence {
                      tunnel: [w255] -> w246
                      tunnel: w242 -> [w255]
                      frame #0 {
                        n131 = Wait (ms)(milliseconds to wait=u32 71000) -> ()  [unwired: 1 out]
                      }
                    }
                  }
                }
                n132 = Unbundle By Name(w108) -> ("status"=w118:bool)
                n133 = Merge Errors(w108, w99) -> (w112:errorcluster)
                n134 = Select(t="TEST", s=w118, f="Espera") -> (s? t:f=w117:string)
                "Path_Borrar" <- path "c:/Trenes" ("file path (use dialog)")
                "Path TEST" <- path "c:/TEST" ("file path (use dialog)")
                "TAGS leidos" <- path "c:/RFID/TAGS.csv" ("file path (use dialog)")
              }
            }
            n135 = call <vilib>:"Watchdog Clear.vi"("error in (no error)"=w90, "watchdogID in"=w91) -> ("error out"=w89:errorcluster)  [unwired: 5 in]
            "Watchdog config" <- w83
          }
          frame "Espera" {
            n136 = local read "Watchdog config"() -> (w262:T3)
            n137 = xnode "Invoke Method"("FPGA VI Reference In"=w274, "error in"=w272) -> ("FPGA VI Reference Out"=w273:refnum<k20>, "error out"=w271:errorcluster)  [unwired: 1 in]
            n138 = local read "Inicio pasada"() -> (w278:timestamp)
            n139 = call <vilib>:"Watchdog Configure.vi"("error in (no error)"=w268, "expiration actions"=w262, "timeout (1 sec)"=3.0) -> ("error out"=w267:errorcluster, "watchdogID"=w266:u64)  [unwired: 1 in, 2 out]
            n140 = while {
              tunnel: [w301] -> w277
              shift-right: [w289] -> w258
              shift-left: w273 -> [w303]
              shift-right: [w288] -> w259
              shift-left: w271 -> [w302]
              tunnel: w278 -> [w306]
              tunnel: w267 -> [w286]
              tunnel: w266 -> [w287]
              tunnel: [w285] -> w265
              tunnel: [w284] -> w264
              i -> [w282]
              stop <- w329 stop-if-true
              # "Modificar F con\nfuente enchufada"
              # "Unir a detector de presencia,\nquitar fotocelula"
              # "El watchdog reinicia el sistema cuando las iteraciones tardan más de x segundo en este bucle"
              n141 = local read "RFID_Error"() -> (w309:errorcluster)
              n142 = disable-structure shown="Disabled" {
                frame Disabled {
                  n143 = call <vilib>:"RT LEDs.vi"("State"=1, "LED Num"=0) -> ()  [unwired: 1 in, 5 out]
                }
                frame Enabled {
                }
              }
              n144 = call <vilib>:"Watchdog Whack.vi"("error in (no error)"=w286, "reset watchdog after expire? (F)"=TRUE, "watchdogID in"=w287) -> ("error out"=w284:errorcluster, "watchdogID out"=w285:u64)  [unwired: 2 in, 1 out]
              n145 = xnode "Read/Write Control"("FPGA VI Reference In"=w303, "error in"=w302) -> ("FPGA VI Reference Out"=w320:refnum<k20>, "error out"=w319:errorcluster, "DC OK"=w324:bool)
              n146 = Unbundle By Name(w309) -> ("status"=w307:bool)
              n147 = call "ControlFuente.vi"("DC OK 3"=w324) -> ("DC OK 2"=→"Fuente":bool, "DC OK"=→"DC OK":string)  [unwired: 1 out]
              n148 = Not(x=w307) -> (.not. x?=→"RFID":bool)
              n149 = xnode "Read/Write Control"("FPGA VI Reference In"=w320, "error in"=w319) -> ("FPGA VI Reference Out"=w315:refnum<k20>, "error out"=w314:errorcluster, "Chassis Temperature"=w322:i16)
              n150 = call "ControlFotocelula_V1.vi"("Tiempo de entrada a espera"=w306) -> ("Aviso no detección"=→"Aviso no detección":string, "Boolean"=w312:bool)
              "Fallo fotocelula" <- w312
              n151 = call "ControlTemperatura.vi"("Chassis Temperature"=w322) -> ("Aviso temperatura"=→"Aviso temperatura":string, "Boolean"=w316:bool, "T fuera rango"=→"T fuera rango":bool)
              n152 = xnode "Read/Write Control"("FPGA VI Reference In"=w315, "error in"=w314) -> ("FPGA VI Reference Out"=w305:refnum<k20>, "error out"=w304:errorcluster, "Detector de presencia"=w296:bool, "RuedaDetectada1?"=→"RuedaDetectada1?":bool, "RuedaDetectada2?"=→"RuedaDetectada2?":bool)
              n153 = Get Date/Time In Seconds() -> (seconds since 1Jan1904=w298:timestamp)
              n154 = Format Date/Time String(seconds (now)=w298, UTC format=FALSE) -> (date/time string=→"date/time string":string)  [unwired: 1 in]
              n155 = Compound Arithmetic op=OR(w316, FALSE ("value"), w312) -> (w313:bool)
              n156 = Compound Arithmetic op=OR("Parar la aplicación", "Reset del controlador", "Configuración") -> (w310:bool)
              n157 = xnode "Read/Write Control"("FPGA VI Reference In"=w305, "error in"=w304, "Fotocélula"="Adquirir") -> ("FPGA VI Reference Out"=w289:refnum<k20>, "error out"=w288:errorcluster)
              n158 = Compound Arithmetic op=OR("Adquirir", w313, w310, w296) -> (w329:bool)
              n159 = Select(t="TEST", s=w313, f="Adquisición") -> (s? t:f=w325:string)
              n160 = Select(t="Configuración", s=w310, f=w325) -> (s? t:f=w301:string)
              "Bucle Espera" <- w282
              "Boton Adquirir?" <- "Adquirir"
            }
            n161 = call <vilib>:"Watchdog Clear.vi"("error in (no error)"=w264, "watchdogID in"=w265) -> ("error out"=w263:errorcluster)  [unwired: 5 in]
            n162 = xnode "Read/Write Control"("FPGA VI Reference In"=w258, "error in"=w259) -> ("FPGA VI Reference Out"=w257:refnum<k20>, "error out"=w256:errorcluster, "Direccion 0?"=→"Direccion 0?":bool)
            n163 = Unbundle By Name(w256) -> ("status"=w276:bool)
            n164 = Select(t="TEST", s=w276, f=w277) -> (s? t:f=w270:string)
            n165 = flat-sequence {
              tunnel: [w280] -> w269
              tunnel: w270 -> [w280]
              frame #0 {
                n166 = Get Date/Time In Seconds() -> (seconds since 1Jan1904=w281:timestamp)
                n167 = To Double Precision Float(number=w281) -> (double precision float=→"Tiempo":dbl)
              }
            }
          }
          frame "Adquisición" {
            n168 = local read "Watchdog config"() -> (w342:T3)
            n169 = call <vilib>:"Watchdog Configure.vi"("error in (no error)"=w341, "expiration actions"=w342, "timeout (1 sec)"=200.0) -> ("error out"=w339:errorcluster, "watchdogID"=w340:u64)  [unwired: 1 in, 2 out]
            n170 = flat-sequence {
              tunnel: w366 -> [w395]
              tunnel: w367 -> [w396]
              tunnel: [w394] -> w356
              tunnel: [w393] -> w355
              tunnel: [w392] -> w354
              tunnel: [w391] -> w353
              tunnel: [w390] -> w352
              tunnel: [w389] -> w351
              tunnel: [w378] -> w344
              tunnel: w340 -> [w377]
              tunnel: w339 -> [w376]
              tunnel: [w377] -> w338
              tunnel: [w376] -> w337
              tunnel: [w411] -> w365
              tunnel: [w428] -> w364
              tunnel: [w427] -> w363
              tunnel: [w426] -> w362
              tunnel: [w419] -> w361
              tunnel: w356 -> [w425]
              tunnel: w355 -> [w424]
              tunnel: w354 -> [w423]
              tunnel: w353 -> [w422]
              tunnel: w352 -> [w421]
              tunnel: w351 -> [w420]
              tunnel: w344 -> [w417]
              tunnel: [w416] -> w343
              tunnel: w338 -> [w415]
              tunnel: w337 -> [w414]
              tunnel: [w412] -> w336
              tunnel: w365 -> [w576]
              tunnel: w364 -> [w571]
              tunnel: w363 -> [w570]
              tunnel: w362 -> [w592]
              tunnel: [w622] -> w348
              tunnel: w361 -> [w624]
              tunnel: [w608] -> w358
              tunnel: [w609] -> w360
              tunnel: [w610] -> w359
              tunnel: w343 -> [w586]
              tunnel: w336 -> [w577]
              tunnel: [w577] -> w334
              tunnel: [w576] -> w333
              frame #0 {
                n171 = local read "Offset_rueda WS 1"() -> (w369:fxp<+/-,24,-4>)
                n172 = local read "Offset_rueda WS 2"() -> (w370:fxp<+/-,24,-4>)
                n173 = local read "Frecuencia de muestreo (Hz)"() -> (w387:dbl)
                n174 = local read "Escaneos de la FIFO por canal"() -> (w375:u32)
                n175 = local read "Canal cero WS1?"() -> (w380:bool)
                n176 = local read "Count(mSec)"() -> (w379:u32)
                n177 = local read "Frecuencia de muestreo y módulo CRIO"() -> (w382:T2)
                n178 = local read "Canal cero WS2"() -> (w368:bool)
                n179 = local read "Digital?"() -> (w381:bool)
                n180 = local read "RFID LR6 on?"() -> (w371:bool)
                n181 = xnode "Read/Write Control"("FPGA VI Reference In"=w396, "error in"=w395, "Data Rate"=w382, "Digital?"=w381, "Canal cero WS1?"=w380, "Count(mSec)"=w379, "Offset_WS1"=w369, "Offset_WS2"=w370, "Canal cero WS2?"=w368) -> ("FPGA VI Reference Out"=w386:refnum<k20>, "error out"=w385:errorcluster)
                n182 = case shown="False" w371 {
                  tunnel: [errorcluster {"status"=FALSE, "code"=0, "source"=""} ("error out") w401] -> w378
                  frame False {
                  }
                  frame True {
                    n183 = local read "RFID_LR6_Error"() -> (w402:errorcluster)
                    n184 = call "LH6HD.vi"("error in (no error)"=w402, "Action"=enum16{"Init", "Start", "Read", "Stop", "Exit"}."Start") -> ("error out"=w401:errorcluster)  [unwired: 8 in, 1 out]
                  }
                }
                n185 = Add(x="Nº inductivos", y="Nº de acelerómetros") -> (x+y=w373:i32)
                n186 = call "DMACalc.vi"("Number of Channels"=w373, "Number of Samples"=w375, "Rate (Hz)"=w387) -> ("Block Size"=w391:u32, "Time to Acquire Block (ms)"=w392:i32, "Host Buffer Size"=w397:u32)  [unwired: 6 in]
                n187 = call "Pathhorafech(SubVI)_varios.vi"("Folder path"=path "c:/Trenes", "Nº de acelerómetros"="Nº de acelerómetros", "Nº inductivos"="Nº inductivos") -> ("Acel_Paths"=w383:path[])  [unwired: 1 in, 1 out]
                "Nombre de archivo" <- w383
                n188 = for {
                  tunnel: w383 -> [w406] mode=indexing
                  tunnel: [w405] -> w390 mode=indexing
                  tunnel: [w404] -> w389
                  n189 = Open/Create/Replace File(file path (use dialog)=w406, operation (0:open)=T6."replace or create", access (0:read/write)=enum16{"read/write", "read-only", "write-only"}."read/write", disable buffering (F)=TRUE) -> (refnum out=w405:refnum<file>, error out=w404:errorcluster)  [unwired: 1 in, 2 out]
                }
                n190 = xnode "Invoke Method"("FPGA VI Reference In"=w386, "error in"=w385, "Requested Depth"=w397) -> ("FPGA VI Reference Out"=w399:refnum<k20>, "error out"=w398:errorcluster)  [unwired: 1 out]
                n191 = Get Date/Time In Seconds() -> (seconds since 1Jan1904=→"Inicio pasada":timestamp)
                n192 = xnode "Invoke Method"("FPGA VI Reference In"=w399, "error in"=w398) -> ("FPGA VI Reference Out"=w394:refnum<k20>, "error out"=w393:errorcluster)
              }
              frame #1 {
                n193 = while "Data Acquisition" {
                  tunnel: w425 -> [w480]
                  shift-right: [w505] -> _
                  shift-left: u32 0 ("t") -> [w501]
                  tunnel: w423 -> [w506]
                  tunnel: w422 -> [w504]
                  shift-right: [w507] -> w427
                  shift-left: w424 -> [w498]
                  tunnel: [w502] -> w428
                  tunnel: w421 -> [w484]
                  tunnel: [w485] -> w426
                  shift-right: [w483] -> w419
                  shift-left: w420 -> [w494]
                  i -> [w479]
                  stop <- w503 stop-if-true
                  # "Detector de presencia"
                  # "Mide el tiempo de paso del tren y con ello se puede calcular\nla velocidad la unidad"
                  n194 = xnode "Invoke Method"("FPGA VI Reference In"=w480, "error in"=w498, "Number of Elements"=w501, "Timeout (ms)"=0) -> ("FPGA VI Reference Out"=w476:refnum<k20>, "error out"=w482:errorcluster, "Data"=w497:fxp<+/-,24,4>[], "Elements Remaining"=w499:u32)
                  n195 = case "Data Ready" shown="Default" w501 {
                    tunnel: w506 -> [w529 _]
                    tunnel: [w528 u32 0 ("t")] -> w505
                    tunnel: w504 -> [w530 _]
                    tunnel: w499 -> [w527 _]
                    tunnel: w497 -> [_ w552]
                    tunnel: w494 -> [w526 w551]
                    tunnel: [w526 w553] -> w483
                    tunnel: w484 -> [w525 w550]
                    tunnel: [w525 w549] -> w485
                    frame 0 {
                      # "En este caso se compara los elementos que quedan\nen la FIFO del controlador con el tamaño dell bloque\nque aparece en el panel frontal. Si el número de \nelementos en la FIFO es mayor o igual que el tamaño\n del bloque se pasa al siguiente caso y se guardan \nlos datos en un archivo. El reloj que aparece es una\nespera para no consumir recursos."
                      n196 = Greater Or Equal?(x=w527, y=w530) -> (x >= y?=w531:bool)
                      n197 = case shown="False" w531 {
                        tunnel: [u32 0 ("Block Size") w535] -> w528
                        tunnel: [w534 0 ("t")] -> w532
                        tunnel: w529 -> [w534 _]
                        tunnel: w530 -> [_ w535]
                        frame False {
                        }
                        frame True {
                        }
                      }
                      n198 = call "WaitMinTimeBetweenCall.vi"("Minimum ms between calls"=w532) -> ()  [unwired: 2 in]
                    }
                    frame Default {
                      n199 = To Single Precision Float(number=w552) -> (single precision float=w539:sgl[])
                      n200 = Decimate 1D Array(w539) -> (w545:sgl[], w548:sgl[], w547:sgl[], w546:sgl[], w544:sgl[], w543:sgl[], w542:sgl[], w541:sgl[], w540:sgl[], w537:sgl[])
                      n201 = Build Array(w545, w548, w547, w546, w544, w543, w542, w541, w540, w537) -> (w538:sgl[][])
                      n202 = for {
                        tunnel: T7."little-endian" ("byte order (0:big-endian, network order)") -> [w562]
                        shift-right: [w556] -> w553
                        shift-left: w551 -> [w557]
                        tunnel: w538 -> [w560] mode=indexing
                        tunnel: w550 -> [w559] mode=indexing
                        tunnel: [w558] -> w549 mode=indexing
                        n203 = Write to Binary File(file (use dialog)=w559, data=w560, error in=w557, 5:FALSE ("prepend array or string size? (T)"), 9:w562) -> (refnum out=w558:refnum<file>, error out=w556:errorcluster)  [unwired: 2 out]
                      }
                    }
                  }
                  n204 = xnode "Read/Write Control"("FPGA VI Reference In"=w476, "error in"=w482) -> ("FPGA VI Reference Out"=w496:refnum<k20>, "error out"=w495:errorcluster, "Parar"=w472:bool, "Nº Ruedas 1"=→"Nº Ruedas 1":i32, "NºRuedas 2"=→"NºRuedas 2":i32)
                  "Parar" <- w472
                  n205 = case shown="False" w472 {
                    tunnel: [w511 w520] -> w473
                    tunnel: [w513 0.0] -> w488
                    frame False {
                      n206 = local read "Inicio pasada"() -> (w516:timestamp)
                      n207 = Get Date/Time In Seconds() -> (seconds since 1Jan1904=w515:timestamp)
                      n208 = To Double Precision Float(number=w515) -> (double precision float=w514:dbl)
                      n209 = To Double Precision Float(number=w516) -> (double precision float=w517:dbl)
                      n210 = Subtract(x=w514, y=w517) -> (x-y=w513:dbl)
                      "Tiempo de paso (s)" <- w513
                      n211 = local write "Tiempo"(w514) -> ()
                      n212 = local read "Boton Adquirir?"() -> (w508:bool)
                      n213 = Greater?(x=w513, y="Tiempo de adquisicion") -> (0:w510:bool)
                      n214 = Select(t=w510, s=w508, f=FALSE) -> (s? t:f=w511:bool)
                    }
                    frame True {
                      n215 = local read "Tiempo"() -> (w524:dbl)
                      n216 = local read "Tiempo extra al detector de paso (s)"() -> (w519:dbl)
                      n217 = Get Date/Time In Seconds() -> (seconds since 1Jan1904=w521:timestamp)
                      n218 = To Double Precision Float(number=w521) -> (double precision float=w522:dbl)
                      n219 = Subtract(x=w522, y=w524) -> (x-y=w523:dbl)
                      "Tiempo extra de adquisición (s)" <- w523
                      n220 = Greater?(x=w523, y=w519) -> (0:w520:bool)
                    }
                  }
                  "Fin" <- w473
                  n221 = local read "Timeout ruedas"() -> (w471:dbl)
                  n222 = xnode ("CheckLate")("FPGA VI Reference In"=w496, "error in"=w495) -> ("FPGA VI Reference Out"=w478:refnum<k20>, "error out"=w491:errorcluster, "Buffer Underflow"=→"Buffer Underflow":bool, "Buffer Overflow"=w481:bool)
                  "Buffer Overflow" <- w481
                  n223 = Greater?(x=w488, y=w471) -> (0:w486:bool)
                  "Timeout ruedas" <- w486
                  n224 = call "ErrorOverFlow.vi"("Buffer Overflow"=w481) -> ("error out"=w489:errorcluster)
                  n225 = call "ErrorUnderFlow.vi"() -> ("error out"=w490:errorcluster)  [unwired: 1 in]
                  n226 = Merge Errors(w491, w490, w489) -> (w477:errorcluster)
                  n227 = Unbundle By Name(w483) -> ("status"=w487:bool)
                  n228 = Unbundle By Name(w477) -> ("status"=w493:bool)
                  n229 = Compound Arithmetic op=OR(w493, w473, w486, w487) -> (w503:bool)
                  "result" <- w503
                  n230 = case "Flush" shown="True" w503 {
                    tunnel: [w563 w568] -> w507
                    tunnel: [w564 w567] -> w502
                    tunnel: w478 -> [w564 w566]
                    tunnel: w477 -> [w563 w565]
                    frame False {
                    }
                    frame True {
                      n231 = xnode "Invoke Method"("FPGA VI Reference In"=w566, "error in"=w565) -> ("FPGA VI Reference Out"=w567:refnum<k20>, "error out"=w568:errorcluster)
                    }
                  }
                  "Block Size" <- w504
                  "Time to Acquire Block (ms)" <- w506
                  "Numeric 3" <- w479
                }
                n232 = call <vilib>:"Watchdog Whack.vi"("error in (no error)"=w414, "reset watchdog after expire? (F)"=TRUE, "watchdogID in"=w415) -> ("error out"=w411:errorcluster, "watchdogID out"=w412:u64)  [unwired: 2 in, 1 out]
                n233 = local read "RFID LR6 on?"() -> (w410:bool)
                n234 = case shown="True" w410 {
                  tunnel: w417 -> [w429 w435]
                  tunnel: [w429 w434] -> w416
                  frame False {
                  }
                  frame True {
                    n235 = while {
                      shift-right: [w442] -> w434
                      shift-left: w435 -> [w443]
                      shift-right: [w441] -> w432
                      shift-left: string[] [] -> [w440]
                      shift-right: [w436] -> w430
                      shift-left: i32[] [] -> [w437]
                      i -> [w438]
                      stop <- w439 stop-if-true
                      n236 = case shown="No Error" w443 {
                        selector: w443 -> [w454 _]
                        tunnel: [w453 w469] -> w442
                        tunnel: [w449 string[] []] -> w441
                        tunnel: w440 -> [w448 _]
                        tunnel: w438 -> [w447 _]
                        tunnel: w437 -> [w446 _]
                        tunnel: [w445 i32[] []] -> w436
                        frame No Error {
                          n237 = call "LH6HD.vi"("error in (no error)"=w454, "Action"=enum16{"Init", "Start", "Read", "Stop", "Exit"}."Read") -> ("error out"=w453:errorcluster, "Tag"=w450:string)  [unwired: 8 in]
                          n238 = Not Equal?(x="", y=w450) -> (x != y?=w451:bool)
                          n239 = case shown="False" w451 {
                            tunnel: w450 -> [_ w463]
                            tunnel: [w457 w462] -> w449
                            tunnel: w448 -> [w457 w461]
                            tunnel: w447 -> [_ w458]
                            tunnel: w446 -> [w456 w460]
                            tunnel: [w456 w459] -> w445
                            frame False {
                            }
                            frame True {
                              n240 = Build Array (concatenate)(w461, w463) -> (w462:string[])
                              n241 = Build Array (concatenate)(w460, w458) -> (w459:i32[])
                            }
                          }
                        }
                        frame Error {
                          n242 = local read "LR6 IP address"() -> (w466:string)
                          n243 = local read "DeviceAddress"() -> (w464:u8)
                          n244 = local read "Port LR6"() -> (w467:u16)
                          n245 = call "LH6HD.vi"("DeviceAddress"=w464, "Reader Port"=w467, "IP Address"=w466, "Action"=enum16{"Init", "Start", "Read", "Stop", "Exit"}."Init") -> ("error out"=w469:errorcluster)  [unwired: 6 in, 1 out]
                        }
                      }
                      n246 = Wait Until Next ms Multiple(millisecond multiple=u32 500) -> ()  [unwired: 1 out]
                      n247 = local read "result"() -> (w439:bool)
                      "it-LR6" <- w438
                    }
                    "TAGs LR6" <- w432
                    "it-read-LR6" <- w430
                  }
                }
              }
              frame #2 {
                n248 = local read "RFID LR6 on?"() -> (w572:bool)
                n249 = Array Size(array=w592) -> (size(s)=w590:i32)
                n250 = local read "TAGs LR6"() -> (w579:string[])
                n251 = local read "timeout ms (60000)"() -> (w575:i32)
                n252 = local read "bytes to read"() -> (w574:i32)
                n253 = local read "RFID NEM on?"() -> (w573:bool)
                n254 = Decrement(x=w590) -> (x-1=w591:i32)
                n255 = local read "Puerto RFID"() -> (w607:u16)
                n256 = case shown="False" w572 {
                  tunnel: w586 -> [w632 w634]
                  tunnel: [w632 w633] -> w585
                  frame False {
                  }
                  frame True {
                    n257 = call "LH6HD.vi"("error in (no error)"=w634, "Action"=enum16{"Init", "Start", "Read", "Stop", "Exit"}."Stop") -> ("error out"=w633:errorcluster)  [unwired: 8 in, 1 out]
                  }
                }
                n258 = local read "RFID_Error"() -> (w618:errorcluster)
                n259 = local read "IP RFID"() -> (w589:string)
                n260 = local read "RFID_ID"() -> (w617:refnum<k5>)
                n261 = Index Array(array=w592, index=w591) -> (element=w600:refnum<file>)
                n262 = local write "result"(FALSE ("result")) -> ()
                n263 = case shown="True" w573 {
                  tunnel: [_ w647] -> w619
                  tunnel: w618 -> [w637 w646]
                  tunnel: w617 -> [w636 w645]
                  tunnel: [w636 w644] -> w616
                  tunnel: [w637 w643] -> w611
                  tunnel: w607 -> [_ w642]
                  tunnel: w589 -> [_ w641]
                  tunnel: [_ w640] -> w569
                  tunnel: w575 -> [_ w639]
                  tunnel: w574 -> [_ w638]
                  frame False {
                  }
                  frame True {
                    n264 = call "RFID_28_03_12.vi"("BYTES TO READ"=w638, "TIMEOUT"=w639, "RFID_Error"=w646, "Puerto RFID"=w642, "IP RFID"=w641, "RFID ID"=w645) -> ("RFID Error"=w643:errorcluster, "connection ID out"=w644:refnum<k5>, "TAGs HEX"=w640:string[], "Unidad"=w647:u32)  [unwired: 1 in]
                  }
                }
                "TAGs HEX" <- w569
                n265 = local write "RFID_LR6_Error"(w585) -> ()
                n266 = for {
                  tunnel: w579 -> [w650] mode=indexing
                  tunnel: [w648] -> w578 mode=indexing
                  n267 = Search and Replace String(input string=w650, search string="00") -> (result string=w648:string)  [unwired: 6 in, 3 out]
                }
                n268 = xnode "Read/Write Control"("FPGA VI Reference In"=w571, "error in"=w570) -> ("FPGA VI Reference Out"=w621:refnum<k20>, "error out"=w620:errorcluster, "Chassis Temperature"=w630:i16)
                n269 = Index Array(array=w569) -> (element=w584:string)  [unwired: 1 in]
                n270 = Not Equal?(x=w584, y="" ("delimiter (\\t)")) -> (x != y?=w582:bool)
                "Plataformas?" <- w582
                n271 = case shown="True" w582 {
                  tunnel: w578 -> [w651 w652]
                  tunnel: [w651 w654] -> w587
                  tunnel: w569 -> [_ w653]
                  frame False {
                  }
                  frame True {
                    n272 = call "Union_TAGs_RFIDs.vi"("TAGs LR6"=w652, "TAGs HEX"=w653) -> ("TAGs"=w654:string[])
                  }
                }
                "TAGs" <- w587
                n273 = Divide(x=w630, y=4.0) -> (x/y=w631:dbl)
                "Temperatura (ºC)" <- w631
                n274 = local read "Tiempo de paso (s)"() -> (w614:dbl)
                n275 = local read "Nombre de archivo"() -> (w599:path[])
                n276 = Multiply(x=w614, y=1000.0) -> (x*y=w612:dbl)
                n277 = for {
                  shift-right: [w660] -> w605
                  shift-left: string[] [] -> [w659]
                  tunnel: w587 -> [w658] mode=indexing
                  n278 = Insert Into Array(array=w659, new element=w658) -> (w660:string[])  [unwired: 1 in]
                }
                n279 = Build Array(w631, w612, w619) -> (w625:dbl[])
                n280 = local write "RFID_ID"(w616) -> ()
                n281 = local write "RFID_Error"(w611) -> ()
                n282 = Delete From Array(array=w599) -> (deleted portion=w598:path)  [unwired: 2 in, 1 out]
                n283 = To Single Precision Float(number=w625) -> (single precision float=w628:sgl[])
                n284 = xnode "Read/Write Control"("FPGA VI Reference In"=w621, "error in"=w620, "Stop"=TRUE ("stop")) -> ("FPGA VI Reference Out"=w602:refnum<k20>, "error out"=w601:errorcluster)
                n285 = Path To String(path=w598) -> (string=w604:string)
                n286 = Write to Binary File(file (use dialog)=w600, data=w628, error in=w624, 5:FALSE ("prepend array or string size? (T)"), 9:T7."little-endian" ("byte order (0:big-endian, network order)")) -> (error out=w597:errorcluster)  [unwired: 3 out]
                n287 = local read "Timeout ruedas"() -> (w615:bool)
                n288 = Build Array (concatenate)(w604, w605) -> (w580:string[])
                n289 = local read "TAGS leidos"() -> (w593:path)
                n290 = for {
                  shift-right: [w657] -> w608
                  shift-left: w597 -> [w656]
                  tunnel: w592 -> [w655] mode=indexing
                  n291 = Close File(refnum=w655, error in=w656) -> (error out=w657:errorcluster)  [unwired: 1 out]
                }
                n292 = xnode "Invoke Method"("FPGA VI Reference In"=w602, "error in"=w601) -> ("FPGA VI Reference Out"=w610:refnum<k20>, "error out"=w609:errorcluster)
                n293 = call-poly <vilib>:"Write Delimited Spreadsheet.vi"("file path (dialog if empty)"=w593, "1D data"=w580, "append to file? (F)"=TRUE ("transpose? (no:F)"), "transpose? (F)"=TRUE ("append to file? (new file:F)"), "delimiter (\\t)"=";" ("delimiter (\\t)")) -> ()  [unwired: 9 in, 2 out]
                n294 = Select(t="TEST", s=w615, f="Procesado") -> (s? t:f=w622:string)
              }
            }
            n295 = call <vilib>:"Watchdog Clear.vi"("error in (no error)"=w333, "watchdogID in"=w334) -> ("error out"=w335:errorcluster)  [unwired: 5 in]
            n296 = Unbundle By Name(w360) -> ("status"=w349:bool)
            n297 = Unbundle By Name(w358) -> ("status"=w350:bool)
            n298 = Merge Errors(w358, w335) -> (w357:errorcluster)
            n299 = Compound Arithmetic op=OR(w349, w350) -> (w347:bool)
            n300 = Select(t="TEST", s=w347, f=w348) -> (s? t:f=w345:string)
          }
          frame "Procesado" {
            n301 = local read "Watchdog config"() -> (w667:T3)
            n302 = call <vilib>:"Watchdog Configure.vi"("error in (no error)"=w670, "expiration actions"=w667, "timeout (1 sec)"=300.0) -> ("error out"=w669:errorcluster, "watchdogID"=w666:u64)  [unwired: 1 in, 2 out]
            n303 = flat-sequence {
              tunnel: w669 -> [w692]
              tunnel: [w695] -> w672
              tunnel: w666 -> [w687]
              tunnel: [w686] -> w665
              tunnel: [w685] -> w664
              tunnel: [w900] -> w682
              tunnel: w672 -> [w900]
              tunnel: [w894] -> w663
              tunnel: w665 -> [w894]
              tunnel: [w893] -> w662
              tunnel: w664 -> [w893]
              frame #0 {
                n304 = flat-sequence {
                  tunnel: [w766] -> w694
                  tunnel: [w751] -> w693
                  tunnel: w692 -> [w716]
                  tunnel: [w754] -> w691
                  tunnel: [w741] -> w688
                  tunnel: [w753] -> w690
                  tunnel: [w740] -> w689
                  tunnel: w687 -> [w717]
                  tunnel: [w714] -> w686
                  tunnel: [w713] -> w685
                  frame #0 {
                    # "No es necesario leer el segundo archivo"
                    # "Distancia de\nla unidad"
                    n305 = local read "Nombre de archivo"() -> (w707:path[])
                    n306 = local read "Tabla_flota"() -> (w750:string[][])
                    n307 = call <vilib>:"Watchdog Whack.vi"("error in (no error)"=w716, "reset watchdog after expire? (F)"=TRUE, "watchdogID in"=w717) -> ("error out"=w713:errorcluster, "watchdogID out"=w714:u64)  [unwired: 2 in, 1 out]
                    n308 = local read "TAGs"() -> (w744:string[])
                    n309 = call "Series_ejes_flota.vi"("Tabla_flota"=w750, "Tags"=w744) -> ("Nº Ejes"=w706:i32[], "Series del convoy"=w743:string[])  [unwired: 2 in, 1 out]
                    "Nº Ejes" <- w706
                    n310 = local read "Puntos medios de las ventanas"() -> (w752:dbl[][])
                    n311 = Array Size(array=w707) -> (size(s)=w760:i32)
                    n312 = Add Array Elements(numeric array=w706) -> (sum=w712:i32)
                    "Ejes_convoy" <- w712
                    n313 = Subtract(x=w760, y=2 ("length")) -> (x-y=w762:i32)
                    n314 = Array Size(array=w743) -> (size(s)=→"Nº UTs":i32)
                    n315 = Delete From Array(array=w707, length=2, index=w762) -> (deleted portion=w730:path[], array with subset deleted=w753:path[])
                    n316 = Index Array(array=w730) -> (element #1=w708:path, element #2=w709:path)  [unwired: 2 in]
                    n317 = local read "Frecuencia de muestreo (Hz)"() -> (w697:dbl)
                    n318 = Read from Binary File(5:sgl 0.0, 9:T7."little-endian" ("byte order (0:big-endian, network order)"), 10:-1 ("count (1)"), 11:w709) -> (0:w758:errorcluster, 2:w732:sgl[], 3:w759:refnum<file>)  [unwired: 1 in, 2 out]
                    n319 = local read "Series_flota"() -> (w749:string[])
                    n320 = local read "Offset_rueda WS 2"() -> (w698:fxp<+/-,24,-4>)
                    n321 = Close File(refnum=w759, error in=w758) -> (error out=w754:errorcluster)  [unwired: 1 out]
                    n322 = Read from Binary File(5:sgl 0.0, 9:T7."little-endian" ("byte order (0:big-endian, network order)"), 10:-1 ("count (1)"), 11:w708) -> (0:w728:errorcluster, 2:w720:sgl[], 3:w729:refnum<file>)  [unwired: 1 in, 2 out]
                    n323 = Array Size(array=w732) -> (size(s)=w748:i32)
                    n324 = Close File(refnum=w729, error in=w728) -> ()  [unwired: 2 out]
                    n325 = Subtract(x=w748, y=3 ("length")) -> (x-y=w746:i32)
                    n326 = Array Size(array=w720) -> (size(s)=w724:i32)
                    n327 = Delete From Array(array=w732, length=3, index=w746) -> (deleted portion=→"deleted portion":sgl[], array with subset deleted=w704:sgl[])
                    n328 = call "Distancias_ejes_convoy.vi"("Series_flota1"=w743, "Ejes_UT"=w706, "Puntos medios de las ventanas"=w752, "Series_flota"=w749) -> ("Distancias_entre_ejes_convoy"=w751:dbl[])  [unwired: 1 in]
                    n329 = Subtract(x=w724, y=3 ("length")) -> (x-y=w722:i32)
                    n330 = Delete From Array(array=w720, length=3, index=w722) -> (deleted portion=→"deleted portion 2":sgl[], array with subset deleted=w719:sgl[])
                    n331 = call "Analogico_digital.vi"("Array"=w704, "Offset WS"=w698, "Frecuencia muestreo"=w697) -> ("array w/ subset deleted"=w699:sgl[], "Tiempo\npaso"=w696:dbl)  [unwired: 6 in]
                    "Waveform Graph 2" <- w699
                    n332 = call "Puntos medio de pulso.vi"("DI Inductivo"=w699) -> ("Puntos"=w766:sgl[], "Número de ejes"=w733:i32)  [unwired: 1 in]
                    "Número de ejes detectados" <- w733
                    n333 = Build Array(w704, w719) -> (→"Waveform Graph":sgl[][])
                    n334 = local read "it-LR6"() -> (w736:i32)
                    n335 = local read "it-read-LR6"() -> (w737:i32[])
                    n336 = local read "Plataformas?"() -> (w735:bool)
                    n337 = local read "TAGs"() -> (w739:string[])
                    n338 = local read "TAGs LR6"() -> (w738:string[])
                    n339 = Decrement(x=w733) -> (x-1=w765:i32)
                    n340 = disable-structure shown="Enabled" {
                      disable-tunnel: w704 -> [w775 w778]
                      disable-tunnel: [FALSE ("element") TRUE ("element")] -> w701
                      disable-tunnel: [w769 w777] -> w700
                      frame Disabled {
                        n341 = Equal?(x=w775, y=0.0) -> (x = y?=w772:bool[])
                        n342 = Equal?(x=w775, y=1.0) -> (x = y?=w773:bool[])
                        n343 = Or(x=w772, y=w773) -> (x .or. y?=w769:bool[])
                      }
                      frame Enabled {
                        n344 = Greater?(x=w778, y=0.1) -> (0:w777:bool[])
                      }
                    }
                    n345 = call "Calculo_Velocidad.vi"("Tiempo de paso (s)"=w696, "Ejes"=w765, "Puntos iniciales de las ventanas"=w751) -> ("V (m/s)"=→"V (m/s)":dbl, "Longitud de la unidad"=→"Longitud de la unidad":dbl)
                    n346 = call "TAGs_AURAwheel.vi"("Nº Ejes"=w706, "TAGs"=w739, "Ejes_convoy"=w712, "it-LR6"=w736, "TAGs LR6"=w738, "it-read-LR6"=w737, "Plataformas?"=w735) -> ("TAGS_AURA"=→"TAGs_AURAwheel":string[][])  [unwired: 1 in]
                    n347 = Get Volume Info(11:path "c:/" ("path")) -> (1:→"Disco Duro Disponible (bytes)":i64)  [unwired: 1 in, 5 out]
                    n348 = Equal?(x=w712, y=w733) -> (x = y?=w740:bool)
                    n349 = Search 1D Array(1D array=w700, element=w701) -> (index of element=w702:i32)  [unwired: 1 in]
                    n350 = Equal?(x=w702, y=-1) -> (x = y?=w705:bool)
                    n351 = And(x=w740, y=w705) -> (x .and. y?=w741:bool)
                    "Archivo\nvalido?" <- w741
                  }
                }
                n352 = case shown="True" w688 {
                  tunnel: w691 -> [w782 w813]
                  tunnel: [w782 w812] -> w695
                  tunnel: w694 -> [_ w817]
                  tunnel: w693 -> [_ w815]
                  tunnel: w690 -> [_ w816]
                  tunnel: w689 -> [w780 _]
                  frame False {
                    n353 = local read "Nombre de archivo"() -> (w781:path[])
                    n354 = for {
                      tunnel: w781 -> [w784] mode=indexing
                      tunnel: w780 -> [w783]
                      n355 = flat-sequence {
                        tunnel: w784 -> [w794]
                        tunnel: [w794] -> w787
                        tunnel: [w793] -> w786
                        tunnel: w783 -> [w792]
                        tunnel: w787 -> [w801]
                        tunnel: [w800] -> w785
                        tunnel: w786 -> [w800]
                        tunnel: w785 -> [w803]
                        frame #0 {
                          w793 = path "c:/Est_Adq.csv" ("file path (use dialog)")
                          n356 = Path To String(path=w794) -> (string=w795:string)
                          n357 = Select(t="Nº Ejes detectados WS diferente a Nº Ejes TAGs" ("delimiter (\\t)"), s=w792, f="La señal del inductivo no es digital" ("delimiter (\\t)")) -> (s? t:f=w789:string)
                          n358 = Build Array(w795, w789) -> (w788:string[])
                          n359 = call-poly <vilib>:"Write Delimited Spreadsheet.vi"("file path (dialog if empty)"=w793, "1D data"=w788, "append to file? (F)"=FALSE ("transpose? (no:F)"), "transpose? (F)"=TRUE ("append to file? (new file:F)"), "delimiter (\\t)"=";" ("delimiter (\\t)")) -> ()  [unwired: 9 in, 2 out]
                        }
                        frame #1 {
                          n360 = local read "Borrar archivos\nadquisicion con error"() -> (w799:bool)
                          n361 = case shown="True" w799 {
                            tunnel: w801 -> [_ w802]
                            frame False {
                            }
                            frame True {
                              n362 = Delete(path (use dialog)=w802) -> ()  [unwired: 1 in, 6 out]
                            }
                          }
                        }
                        frame #2 {
                          n363 = File/Directory Info(path=w803) -> (size=w806:i64)  [unwired: 1 in, 6 out]
                          n364 = Greater?(x=w806, y=i64 1000000) -> (0:w804:bool)
                          n365 = case shown="True" w804 {
                            tunnel: w803 -> [_ w807]
                            frame False {
                            }
                            frame True {
                              n366 = Delete(path (use dialog)=w807) -> ()  [unwired: 4 in, 3 out]
                            }
                          }
                        }
                      }
                    }
                  }
                  frame True {
                    n367 = flat-sequence {
                      tunnel: w817 -> [w887]
                      tunnel: w816 -> [w884]
                      tunnel: w815 -> [w888]
                      tunnel: [w872] -> w814
                      frame #0 {
                        # "SALIDA \n\nMáximos por rueda inductivo"
                        # "8 acelerómetros"
                        # "Velocidad"
                        n368 = local read "Frecuencia de muestreo (Hz)"() -> (w886:dbl)
                        n369 = local read "Distancia de acelerómetros"() -> (w876:dbl[])
                        n370 = local read "Parámetros acelerómetros"() -> (w883:dbl[])
                        n371 = local read "Número de ejes detectados"() -> (w882:i32)
                        n372 = local read "Distancias generales"() -> (w881:dbl[])
                        n373 = local read "dt RMS"() -> (w885:dbl)
                        n374 = local read "Direccion 0?"() -> (w873:bool)
                        n375 = Index Array(array=w881, index=1) -> (element=w879:dbl)
                        n376 = Select(t=0.0, s=w873, f=w879) -> (s? t:f=w877:dbl)
                        n377 = Subtract(x=w877, y=w876) -> (x-y=w875:dbl[])
                        n378 = Absolute Value(x=w875) -> (abs(x)=w874:dbl[])
                        n379 = call "Procesado_aRMS_BIdirecc.vi"("Paths_canales_aRMS"=w884, "Ejes Procesados"=w882, "Distancias\nacelerometros"=w874, "Distancias generales (m)"=w881, "Distancias centrales de las ruedas\n               configuración (m)"=w888, "Frecuencia de muestreo"=w886, "Parámetros acelerómetros"=w883, "dt RMS 2"=w885, "Puntos"=w887) -> ("Max RMS Ruedas"=w871:dbl[][])  [unwired: 2 in]
                        n380 = Transpose 2D Array(2D array=w871) -> (transposed array=w872:dbl[][])
                        "Max RMS Ruedas" <- w872
                      }
                    }
                    n381 = local read "Use Aura?"() -> (w811:bool)
                    n382 = local read "TAGs_AURAwheel"() -> (w809:string[][])
                    n383 = local read "Nº Ejes"() -> (w808:i32[])
                    n384 = for {
                      tunnel: w811 -> [w822]
                      tunnel: [w821] -> w810 mode=indexing
                      tunnel: w809 -> [w820] mode=indexing
                      shift-right: [w819] -> _
                      shift-left: w814 -> [w823]
                      tunnel: w808 -> [w818] mode=indexing
                      # "dev.api.aurawheel.com"
                      n385 = case shown="True" w822 {
                        tunnel: w823 -> [w824 w836]
                        tunnel: [errorcluster {"status"=FALSE, "code"=0, "source"=""} ("error out") w841] -> w821
                        tunnel: w820 -> [_ w837]
                        tunnel: [w824 w835] -> w819
                        tunnel: w818 -> [_ w833]
                        frame False {
                        }
                        frame True {
                          w845 = cluster{"status":string} {"status"=""}
                          n386 = local read "Parametros AuraWheel"() -> (w870:string[])
                          n387 = Delete From Array(array=w836, length=w833, index (row)=0) -> (deleted portion=w832:dbl[][], array with subset deleted=w835:dbl[][])  [unwired: 1 in]
                          n388 = Get Date/Time In Seconds() -> (seconds since 1Jan1904=w866:timestamp)
                          n389 = Format Date/Time String(time format string (%c)="%H:%M:%S%3u", seconds (now)=w866) -> (date/time string=w864:string)  [unwired: 1 in]
                          n390 = Get Date/Time In Seconds() -> (seconds since 1Jan1904=w840:timestamp)
                          n391 = Scan From String(format string="%d:%d:%f", input string=w864) -> (output 1=w861:i32, output 2=w860:i32, output 3=w858:dbl)  [unwired: 5 in, 3 out]
                          n392 = local read "V (m/s)"() -> (w828:dbl)
                          n393 = local read "Temperatura (ºC)"() -> (w838:dbl)
                          n394 = Multiply(x=w828, y=3.6) -> (x*y=w826:dbl)
                          n395 = Multiply(x=w858, y=1000.0) -> (x*y=w854:dbl)
                          n396 = call "Time_to_ms.vi"("seconds since 1Jan1904"=w840) -> ("Numeric"=w839:dbl)  [unwired: 1 in]
                          n397 = Multiply(x=w860, y=60000) -> (x*y=w855:i32)
                          n398 = Multiply(x=3600000, y=w861) -> (x*y=w856:i32)
                          n399 = Index Array(array=w870) -> (element #1=w831:string, element #2=w830:string, element #3=w829:string)  [unwired: 3 in]
                          n400 = call "aw_WRDCluster_8acel.vi"("Array TAGs"=w837, "Max RMS Ruedas"=w832, "TimeStamp"=w839, "p_sp"=w826, "p_tp"=w838) -> ("JSON cluster"=w867:T9)  [unwired: 1 in]
                          n401 = Compound Arithmetic op=ADD(w856, w855, w854) -> (w853:dbl)
                          n402 = To Variant(anything=w867) -> (Variant=w850:variant)
                          n403 = To Unsigned Long Integer(number=w853) -> (unsigned 32bit integer=w852:u32)
                          n404 = call "gjson_Create.vi"("JSON Object in"=w850) -> ("error out"=w848:errorcluster, "JSON String Out"=w849:string)  [unwired: 9 in]
                          n405 = Number To Decimal String(number=w852) -> (decimal integer string=w851:string)  [unwired: 1 in]
                          n406 = To Variant(anything=w845) -> (Variant=w844:variant)
                          n407 = call "aw_SendData.vi"("pwd"=w831, "x-nem-datetime"=w851, "User"=w830, "error in"=w848, "JSON Object"=w849, "URL"=w829) -> ("error out"=w846:errorcluster, "Response JSON"=w847:string, "Response headers"=→"Response headers":string)  [unwired: 3 in]
                          n408 = call "gjson_Parse.vi"("error in"=w846, "JSON String In"=w847, "JSON Cluster"=w844) -> ("error out"=w842:errorcluster, "JSON Cluster Out"=w843:variant)  [unwired: 7 in]
                          n409 = Variant To Data(error in=w842, type=w845, Variant=w843) -> (data=→"data":cluster{"status":string}, error out=w841:errorcluster)
                          "error AURA" <- w841
                        }
                      }
                    }
                    n410 = Merge Errors(w810, w813) -> (w812:errorcluster)
                  }
                }
              }
              frame #1 {
                n411 = local read "Bytes libre despues de borrar"() -> (w890:u32)
                n412 = local read "Archivo\nvalido?"() -> (w889:bool)
                n413 = local read "Bytes min libre"() -> (w891:u32)
                n414 = local read "Max archivos"() -> (w892:u32)
                n415 = local read "TAGS leidos"() -> (w896:path)
                n416 = File/Directory Info(path=w896) -> (size=w899:i64)  [unwired: 1 in, 6 out]
                n417 = local read "Path TEST"() -> (w895:path)
                n418 = case shown="True" w889 {
                  frame False {
                  }
                  frame True {
                    n419 = local read "Nombre de archivo"() -> (w902:path[])
                    n420 = call "Comprimir_a_1_archivo.vi"("Acel_paths"=w902) -> ("path_Pasada"=→"created path":path)
                  }
                }
                n421 = Greater?(x=w899, y=i64 1000000) -> (0:w897:bool)
                n422 = case shown="True" w897 {
                  tunnel: w896 -> [_ w903]
                  frame False {
                  }
                  frame True {
                    n423 = Delete(path (use dialog)=w903) -> ()  [unwired: 4 in, 3 out]
                  }
                }
                n424 = call "BORRADO_MEJORADO_Gonzalo.vi"("Bytes LIBRE OK"=w890, "Bytes Minimo de Memoria libre"=w891) -> ()  [unwired: 10 in]
                n425 = call "Borrar_carpeta.vi"("Nº Archivos Max"=w892, "Path Carpeta"=w895) -> ()  [unwired: 1 in]
              }
            }
            n426 = call <vilib>:"Watchdog Clear.vi"("error in (no error)"=w662, "watchdogID in"=w663) -> ("error out"=w661:errorcluster)  [unwired: 5 in]
            n427 = local read "RFID_Error"() -> (w673:errorcluster)
            n428 = Merge Errors(w682, w661) -> (w674:errorcluster)
            n429 = Merge Errors(w671, w673, w674) -> (w683:errorcluster)
            n430 = Unbundle By Name(w683) -> ("status"=w677:bool)
            n431 = Select(t="Descarga datos", s=FALSE, f="Espera") -> (s? t:f=w679:string)
            n432 = Select(t="TEST", s=w677, f=w679) -> (s? t:f=w676:string)
          }
          frame "TEST" {
            n433 = local read "Watchdog config"() -> (w912:T3)
            n434 = call <vilib>:"Watchdog Configure.vi"("expiration actions"=w912, "timeout (1 sec)"=200.0) -> ("error out"=w913:errorcluster, "watchdogID"=w910:u64)  [unwired: 2 in, 2 out]
            n435 = flat-sequence {
              tunnel: [w928] -> w917
              tunnel: w913 -> [w923]
              tunnel: w915 -> [w942]
              tunnel: [w941] -> w905
              tunnel: [w924] -> w914
              tunnel: w910 -> [w922]
              tunnel: [w921] -> w908
              tunnel: w909 -> [w920]
              tunnel: [w919] -> w907
              frame #0 {
                n436 = call <vilib>:"Watchdog Whack.vi"("error in (no error)"=w923, "reset watchdog after expire? (F)"=TRUE, "watchdogID in"=w922) -> ("error out"=w919:errorcluster, "watchdogID out"=w921:u64)  [unwired: 2 in, 1 out]
                n437 = Get Date/Time In Seconds() -> (seconds since 1Jan1904=w935:timestamp)
                n438 = local read "Ultimo TEST"() -> (w936:timestamp)
                n439 = To Double Precision Float(number=w935) -> (double precision float=w937:dbl)
                n440 = Subtract(x=w937, y=3600.0) -> (x-y=w939:dbl)
                n441 = To Time Stamp(1:w939) -> (0:w940:timestamp)
                n442 = In Range and Coerce(upper limit=w935, x=w936, lower limit=w940) -> (In Range?=w934:bool)  [unwired: 1 out]
                n443 = case shown="False" w934 {
                  tunnel: w920 -> [w971 _]
                  tunnel: w942 -> [w947 w986]
                  tunnel: [w956 errorcluster {"status"=FALSE, "code"=0, "source"=""} ("error out")] -> w941
                  tunnel: [w947 w986] -> w924
                  frame False {
                    n444 = local read "Timeout ruedas"() -> (w948:bool)
                    n445 = local read "Aviso no detección"() -> (w954:string)
                    n446 = local read "Aviso temperatura"() -> (w953:string)
                    n447 = case shown="True" w948 {
                      selector: w948 -> [_ w983]
                      tunnel: ["\r" w984] -> w946
                      frame False {
                      }
                      frame True {
                        w973 = "\n"
                        n448 = local read "Nº Ruedas 1"() -> (w980:i32)
                        n449 = local read "NºRuedas 2"() -> (w975:i32)
                        n450 = call "ErrorRuedas.vi"("Buffer Overflow"=w983) -> ("error out"=w985:errorcluster)
                        n451 = Number To Decimal String(number=w980) -> (decimal integer string=w978:string)  [unwired: 1 in]
                        n452 = Number To Decimal String(number=w975) -> (decimal integer string=w974:string)  [unwired: 1 in]
                        n453 = Concatenate Strings("Error Wheel sensors", "\n", "WS1 (ruedas):", w978, w973, "WS2 (ruedas):", w974, w973) -> (w976:string)
                        n454 = call "Error.vi"("Error con..."=w976, "error comunicacion 2"=w985) -> ("String"=w984:string)
                      }
                    }
                    n455 = local read "RFID_Error"() -> (w950:errorcluster)
                    n456 = local read "RFID_LR6_Error"() -> (w944:errorcluster)
                    n457 = local read "DC OK"() -> (w952:string)
                    n458 = call "Cabecera.vi"() -> ("String"=w969:string)
                    n459 = call "Adquisicion.vi"("Aviso no detección"=w954) -> ("String"=w968:string)
                    n460 = call "Temperatura.vi"("Aviso temperatura"=w953) -> ("String"=w967:string)
                    n461 = call "Fuente.vi"("DC OK"=w952) -> ("String"=w966:string)
                    n462 = call "FPGA.vi"("error out"=w947) -> ("String"=w965:string)
                    n463 = call "Escritura.vi"("error out"=w971) -> ("String"=w964:string)
                    n464 = call "Error.vi"("Error con..."="Error con el lecto RFID NEM", "error comunicacion 2"=w950) -> ("String"=w949:string)
                    n465 = call "Error.vi"("Error con..."="Error con el lecto RFID LR6-HD", "error comunicacion 2"=w944) -> ("String"=w943:string)
                    n466 = Concatenate Strings(w969, w968, w967, w966, w965, w964, w949, w943, w946) -> (w970:string)
                    n467 = call "STRINGhorafechA(SubVI).vi"() -> ("STRINGhora_fecha"=w963:string)
                    n468 = Concatenate Strings(w963, ".txt" ("string")) -> (w959:string)
                    n469 = Get Date/Time In Seconds() -> (seconds since 1Jan1904=→"Ultimo TEST":timestamp)
                    n470 = Build Array("c", "TEST" ("element"), w959) -> (w961:string[])
                    n471 = Array of Strings to Path(0:w961) -> (2:w957:path)  [unwired: 1 out]
                    n472 = Write to Text File(file (use dialog)=w957, text=w970) -> (error out=w956:errorcluster)  [unwired: 1 in, 3 out]
                  }
                  frame True {
                  }
                }
                n473 = local read "Fallo fotocelula"() -> (w927:bool)
                n474 = Unbundle By Name(w924) -> ("status"=w925:bool)
                n475 = local read "T fuera rango"() -> (w933:bool)
                n476 = Compound Arithmetic op=OR(w925, w927) -> (w926:bool)
                n477 = local write "Reset del controlador"(w926) -> ()
                n478 = Select(t="Escape", s=w933, f="Espera") -> (s? t:f=w930:string)
                n479 = Select(t="Configuracion", s=w926, f=w930) -> (s? t:f=w928:string)
              }
            }
            n480 = call <vilib>:"Watchdog Clear.vi"("error in (no error)"=w907, "watchdogID in"=w908) -> ("error out"=w906:errorcluster)  [unwired: 5 in]
            n481 = Merge Errors(w906, w905) -> (w904:errorcluster)
          }
        }
        "Estado" <- w77
        "error manipulacion archivos" <- w79
        n482 = local read "Parar la aplicación"() -> (w76:bool)
      }
      n483 = xnode "Close FPGA VI Reference"("FPGA VI Reference In"=w69, "error in"=w68) -> ("error out"=→"error FPGA":errorcluster)
    }
    frame #3 {
      n484 = local read "RFID_ID"() -> (w990:refnum<k5>)
      n485 = call "LH6HD.vi"("Action"=enum16{"Init", "Start", "Read", "Stop", "Exit"}."Stop") -> ("error out"=→"RFID_LR6_Error":errorcluster)  [unwired: 9 in, 1 out]
      n486 = TCP Close Connection(connection ID=w990) -> (error out=→"RFID_Error":errorcluster)  [unwired: 1 in, 2 out]
    }
  }
